vi "Teleop.vi"(10 "Match Info":T1={"Autonomous Elapsed Seconds"=0.0, "TeleOp Elapsed Seconds"=0.0, "Disabled Elapsed Seconds"=0.0, "Visited Autonomous"=FALSE, "Visited TeleOp"=FALSE, "Visited Disabled"=FALSE, "Autonomous Settings"={"Autonomous Style"=enum."Independent", "VI Refnum"=refnum}}, 11 "Call Context":T2) -> ()   [LabVIEW 2017]
doc: "This VI is called for each TeleOp packet received from the DS where the robot is not disabled. It is often used to read from the joysticks and update I/O or to update setpoints for timed control loops. It should complete and return within 20 milliseconds or it may miss DS packets."
uses:
  <vilib>/Rock Robotics/WPI/DriverStation/WPI_DriverStationDerivedRobotMode.ctl
  <vilib>/Rock Robotics/WPI/DriverStation/WPI_DriverStationMatch Info.ctl
  Public/Documents/Cross The Road Electronics/Phoenix-LabVIEW/Motor Controller/Controls/CTRE_Phoenix_MotorControl_ControlMode.ctl
  Public/Documents/Cross The Road Electronics/Phoenix-LabVIEW/Motor Controller/Controls/CTRE_Phoenix_MotorControl_FeedbackDevice.ctl
  <vilib>/Rock Robotics/Network Tables/NT Read Boolean.vi
  Public/Documents/Cross The Road Electronics/Phoenix-LabVIEW/Motor Controller/Get/CTRE_Phoenix_MotorController_GetSelectedSensorData.vi
  Public/Documents/Cross The Road Electronics/Phoenix-LabVIEW/Motor Controller/Get/CTRE_Phoenix_MotorController_GetPulseWidthAll.vi
  <vilib>/Utility/config.llb/Write Key (I32).vi
  <vilib>/Rock Robotics/Network Tables/NT Write Boolean.vi
  <vilib>/Utility/config.llb/Read Key (Double).vi
  <vilib>/Rock Robotics/Network Tables/NT Write Number.vi
  <vilib>/Rock Robotics/WPI/Utilities/WPI_GetSetVariantRefNum.vi
  Public/Documents/Cross The Road Electronics/Phoenix-LabVIEW/Motor Controller/Get/CTRE_Phoenix_MotorController_GetQuadratureData.vi
  <vilib>/Rock Robotics/WPI/Solenoid/Deprecated/WPI_SolenoidSetBool.vi
  Public/Documents/Cross The Road Electronics/Phoenix-LabVIEW/Motor Controller/Get/CTRE_Phoenix_MotorController_GetTemperature.vi
  Public/Documents/Cross The Road Electronics/Phoenix-LabVIEW/Motor Controller/Get/CTRE_Phoenix_MotorController_GetOutputCurrent_Enhanced.vi
  Robot Global Data.vi
  <vilib>/Utility/config.llb/NI_LVConfig.lvlib
  <vilib>/ptbypt/NI_PtbyPt.lvlib
panel:
  out "hasSet":bool
  out "ClimberDelay":dbl
  out "Holding Current":dbl=9001.0
  out "Old Direction":bool
  out "Stalled":bool
  out "OutHalf":bool
  out "EndGame":bool
  out "In":bool
  out "Hook":bool
  out "OutFULL":bool
  out "RobotOrientedPos":dbl
  out "RobotOriented":bool
  in  "Elevator Config":dbl(slide) scale=-1.0..1.0
  out "Rotate 3":dbl
  out "Rotate 2":dbl
  out "Rotate 1":dbl
  out "Rotate 0":dbl
  out "Turn3":dbl
  out "Turn2":dbl
  out "Turn1":dbl
  out "Turn0":dbl
  out "Speed0":dbl
  out "Speed1":dbl
  out "Speed2":dbl
  out "Speed3":dbl
  out "max":dbl
  out "angle":dbl
  out "temp":dbl
  out "Y":dbl
  out "X":dbl
  out "C":dbl
  out "D":dbl
  out "B":dbl
  out "A":dbl
  out "R":dbl
  out "W":dbl=22.75
  out "L":dbl=22.25
  out "RCW":dbl
  out "STR":dbl
  out "FWD":dbl
  out "Temp Speed0":dbl
  out "Temp Speed1":dbl
  out "Temp Speed2":dbl
  out "Temp Speed3":dbl
  out "Temp Turn3":dbl
  out "Temp Turn2":dbl
  out "Temp Turn1":dbl
  out "Temp Turn0":dbl
  out "Elevator Set":dbl=400.0
  out "Elevator Up":bool
  out "Elevator Pry":bool
  out "Elevator Middle":bool
  out "Elevator Down":bool
  out "Found 0? 2":bool
  out "Found 1? 2":bool
  out "Found 2? 2":bool
  out "Found 3? 2":bool
  out "Start Pos 7":i32
  out "Start Pos 6":i32
  out "Start Pos 5":i32
  out "Start Pos 4":i32
  in  "Read Button 2":bool
  out "Current Pos 7":i32
  out "Current Pos 6":i32
  out "Current Pos 5":i32
  out "Current Pos 4":i32
  out "Current Pos 3":i32
  out "Current Pos 1":i32
  out "Current Pos 2":i32
  out "Current Pos 0":i32
  out "Found 0?":bool
  out "Found 1?":bool
  out "Found 2?":bool
  out "Found 3?":bool
  in  "Write Button":bool
  out "Start Pos 3":i32
  out "Start Pos 2":i32
  out "Start Pos 1":i32
  out "Start Pos 0":i32
  in  "Read Button":bool
  out "0-4096 2":dbl
  out "Prev Knob Value":dbl
  out "Intake Motor":dbl
  in  "DriveMode":string(combo)="Mike1"
  out "0-4096":dbl
  out "+-180":dbl
  out "DegDir":dbl
  out "Elevator Change":bool
  out "Aquire":bool
  out "ArmLift":dbl
  out "Knob Value":dbl
  out "Arm Position":dbl
  out "Open/Close":bool
  out "Output Current":dbl
  out "Standby":bool
  out "StandbyWait":dbl
  out "Elevator Read":dbl
  out "Zero Gyro":bool
  out "TONY MODE":bool
  out "Direction":dbl
  out "DIAL":dbl
  out "Gyro":dbl
  out "Pos 3":i32
  out "Pos 2":i32
  out "Pos 1":i32
  out "Joystick":dbl
  out "Pos 0":i32
  out "Distance 2 Go":dbl
  out "Magnitude":dbl
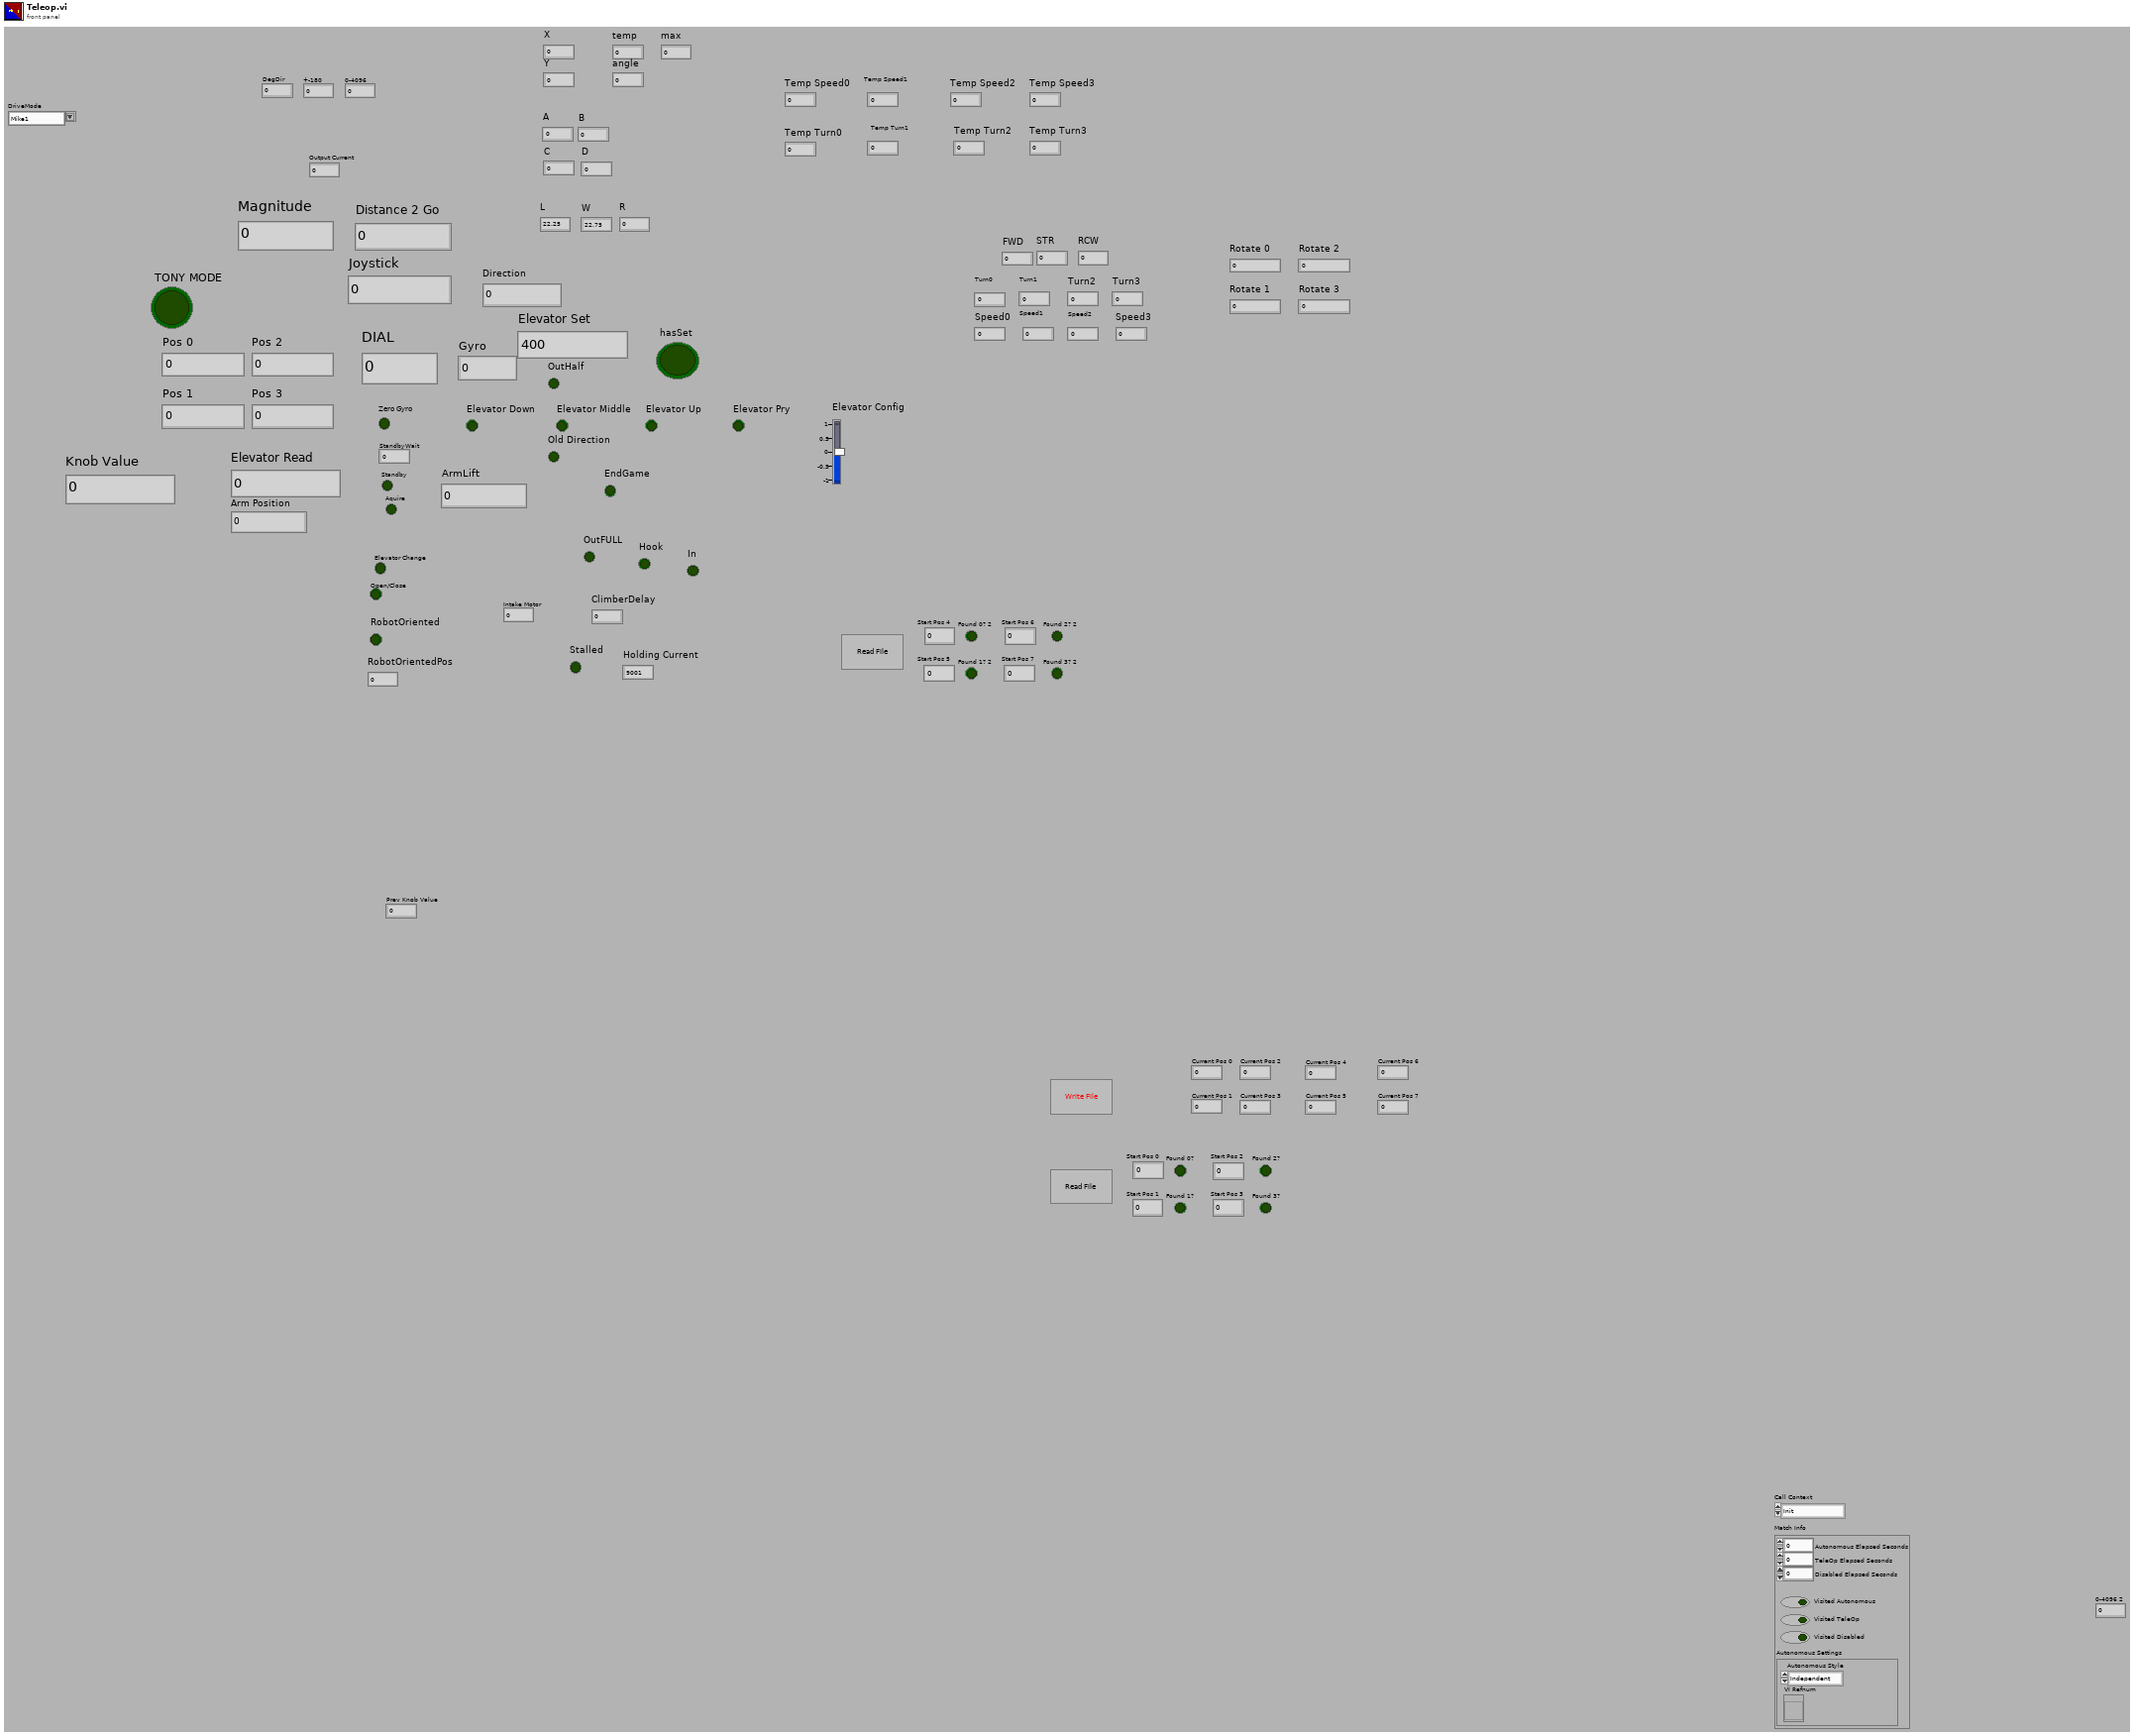
[diagram p1: front panel]
types:
  T1 = typedef "WPI_DriverStationMatch Info.ctl" = cluster{"Autonomous Elapsed Seconds":dbl, "TeleOp Elapsed Seconds":dbl, "Disabled Elapsed Seconds":dbl, "Visited Autonomous":bool, "Visited TeleOp":bool, "Visited Disabled":bool, "Autonomous Settings":cluster{"Autonomous Style":enum16{"Iterative", "Independent"}, "VI Refnum":refnum<vi>}}
  T2 = typedef "WPI_DriverStationDerivedRobotMode.ctl" = enum16{"Init", "Execute", "Stop"}
  T3 = typedef "CTRE_Phoenix_MotorControl_ControlMode.ctl" = u16
  T4 = typedef "WPI_MotorControlDeviceRef.ctl" = cluster{"DeviceStatus":errorcluster, "Type":T5, "PWM":cluster{"PWM Channel":T6, "DeadBand":T7}, "CAN":cluster{"Device Number":u8, "SetOutput VI Ref":variant, "GetOutput VI Ref":variant, "Enable VI Ref":variant, "Disable VI Ref":variant, "Data":variant}, "Invert":bool, "DIO PWM":cluster{"PWM \"Enable\" Channel":T6, "DIOChannel":T8, "PWM Rate":dbl}}
  T5 = typedef "WPI_MotorControlType.ctl" = enum16{"PWM", "CAN", "DIO PWM"}
  T6 = typedef "FPGA_DIOPWMChannel.ctl" = enum8{"PWM 0", "PWM 1", "PWM 2", "PWM 3", "PWM 4", "PWM 5", "PWM 6", "PWM 7", "PWM 8", "PWM 9", "PWM MXP 0", "PWM MXP 1", "PWM MXP 2", "PWM MXP 3", "PWM MXP 4", "PWM MXP 5", "PWM MXP 6", "PWM MXP 7", "PWM MXP 8", "PWM MXP 9", "Invalid"}
  T7 = typedef "WPI_PWMDeadband.ctl" = cluster{"Name":string, "maxPositivePwm":i32, "minPositivePwm":i32, "centerPwm":i32, "maxNegativePwm":i32, "minNegativePwm":i32, "angularRange":u16}
  T8 = typedef "FPGA_DIOChannel.ctl" = enum8{"DIO 0", "DIO 1", "DIO 2", "DIO 3", "DIO 4", "DIO 5", "DIO 6", "DIO 7", "DIO 8", "DIO 9", "DIO MXP 0", "DIO MXP 1", "DIO MXP 2", "DIO MXP 3", "DIO MXP 4", "DIO MXP 5", "DIO MXP 6", "DIO MXP 7", "DIO MXP 8", "DIO MXP 9", "DIO MXP 10", "DIO MXP 11", "DIO MXP 12", "DIO MXP 13", "DIO MXP 14", "DIO MXP 15", "SPI Port CS1", "SPI Port CS2", "SPI Port CS3", "SPI Port MISO", "SPI Port MOSI", "Invalid"}
  T9 = typedef "CTRE_Phoenix_MotorControl_FeedbackDevice.ctl" = i8
  T10 = typedef "NI_LVConfig.lvlib/Config Data RefNum.ctl" = refnum<k1>
  T11 = typedef "WPI_JoystickDevRef.ctl" = cluster{"Device":T12}
  T12 = typedef "WPI_JoystickDeviceEnum.ctl" = enum16{"USB 0", "USB 1", "USB 2", "USB 3", "USB 4", "USB 5"}
  T13 = typedef "WPI_CompressorDevRef.ctl" = cluster{"DevStatus":errorcluster, "Pneumatics Control Module":u8}
  T14 = typedef "WPI_SolenoidDevRef.ctl" = cluster{"DevStatus":errorcluster, "Pneumatics Control Module":u8, "Forward Solenoid Channel":T15, "Reverse Solenoid Channel":T15}
  T15 = typedef "WPI_SolenoidChannel.ctl" = enum8{"Solenoid 0", "Solenoid 1", "Solenoid 2", "Solenoid 3", "Solenoid 4", "Solenoid 5", "Solenoid 6", "Solenoid 7", "Invalid"}
  T16 = typedef "WPI_GyroDevRef.ctl" = cluster{"DevStatus":errorcluster, "Analog Channel":T17, "Gain (VoltsPerDegree/Second)":dbl, "Gyro Type":enum16{"Analog", "XRS450"}, "Handle":i32, "SPI Bus":T18, "Device Found":bool, "Sample Rate":dbl, "Calibrate On Open":bool, "Offset":dbl}
  T17 = typedef "FPGA_AIChannel.ctl" = enum8{"AI 0", "AI 1", "AI 2", "AI 3", "AI MXP 0", "AI MXP 1", "AI MXP 2", "AI MXP 3", "Invalid"}
  T18 = typedef "spi_bus.ctl" = enum16{"SPI On-Board, CS0", "SPI On-Board, CS1", "SPI On-Board, CS2", "SPI On-Board, CS3", "SPI MXP", "Invalid"}
  T19 = typedef "WPI_DigitalInputDevRef.ctl" = cluster{"DevStatus":errorcluster, "DIO Channel":T8}
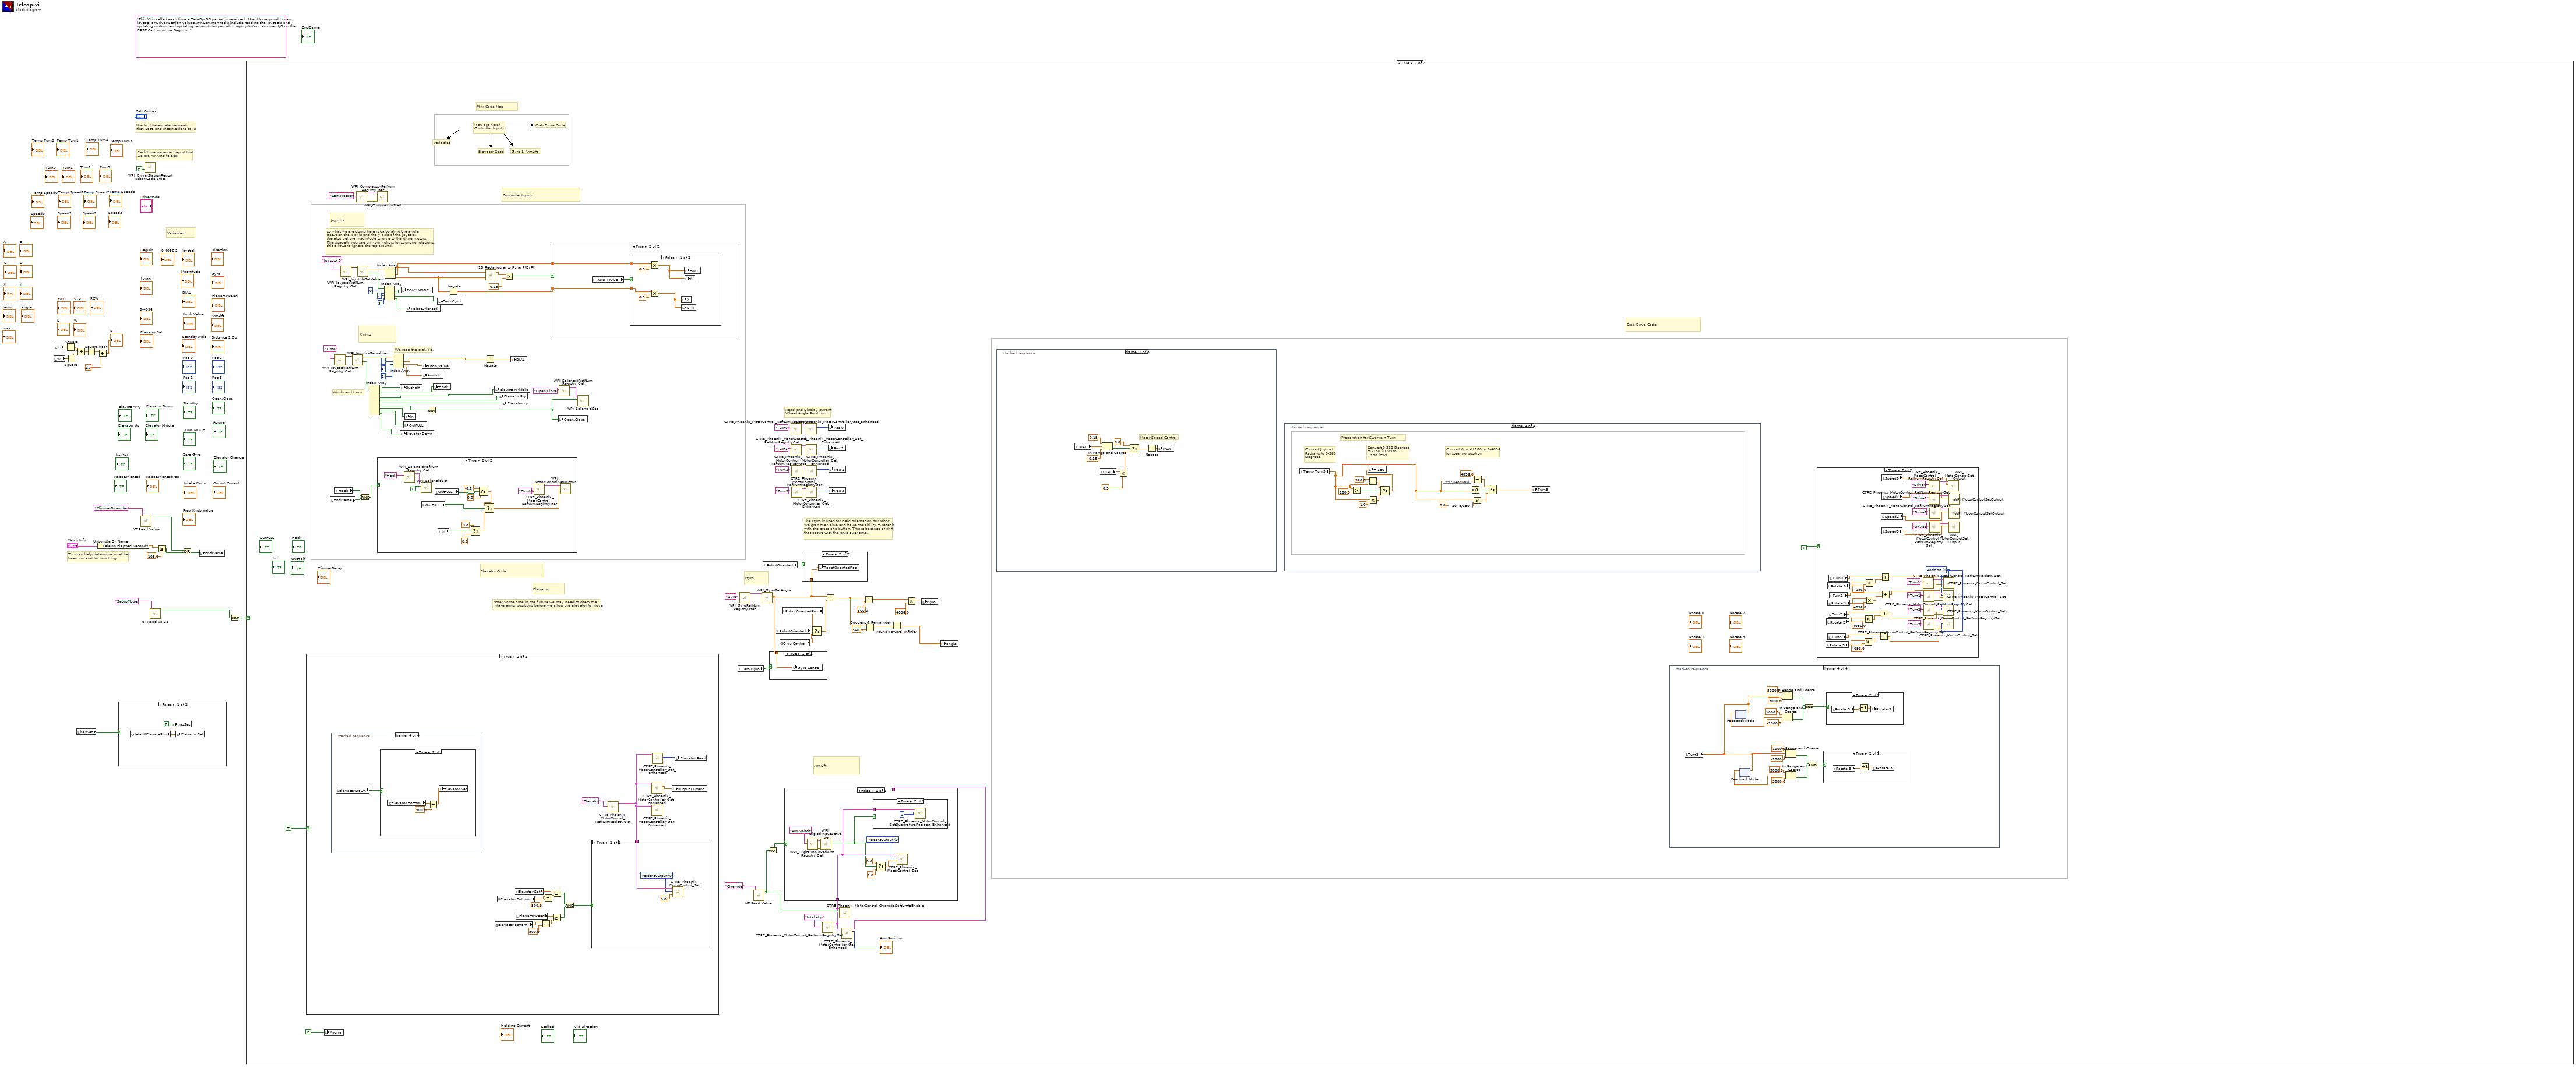
[diagram p0: block diagram]
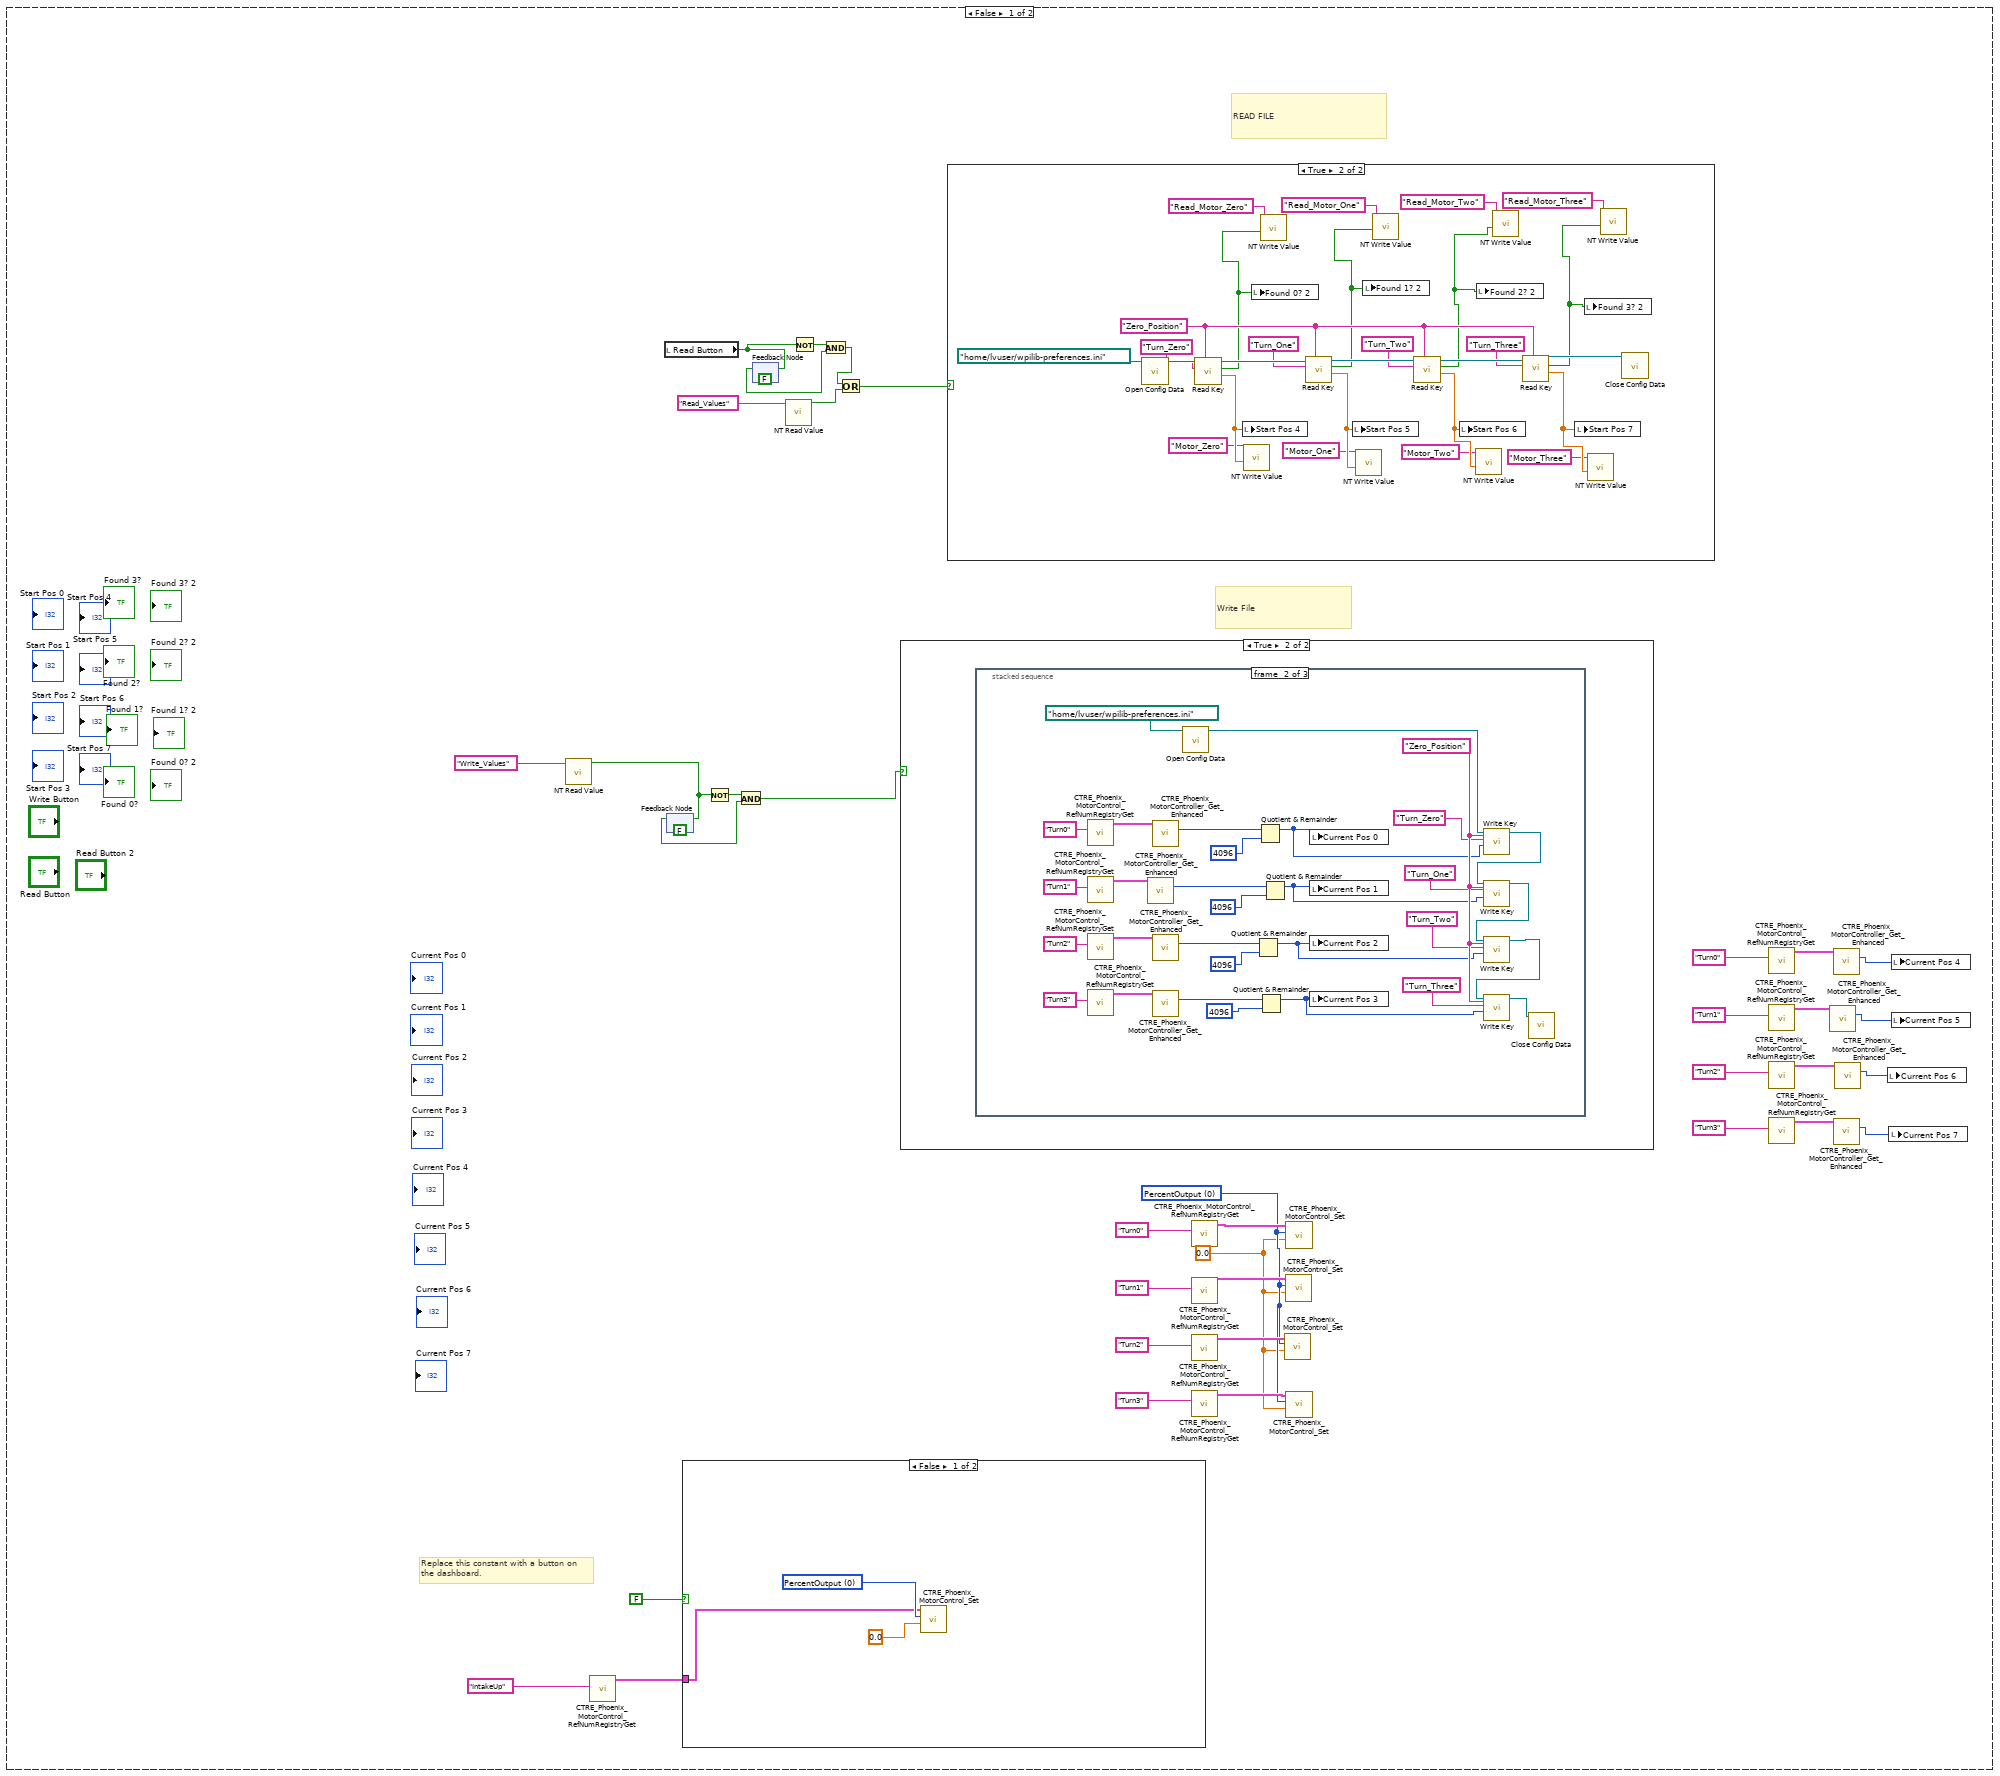
[diagram p3: hidden frame]
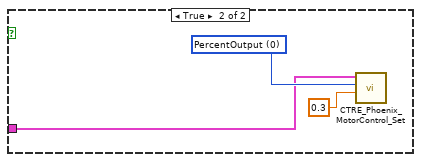
[diagram p4: hidden frame]
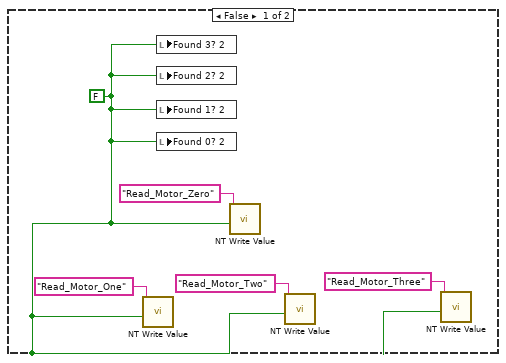
[diagram p5: hidden frame]
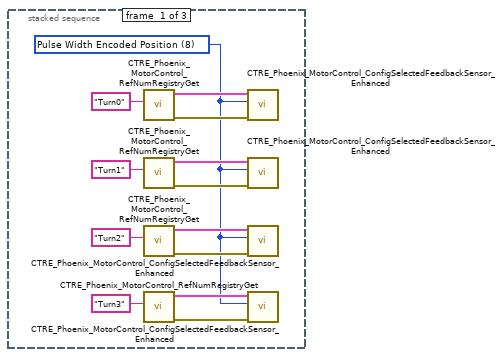
[diagram p7: hidden frame]
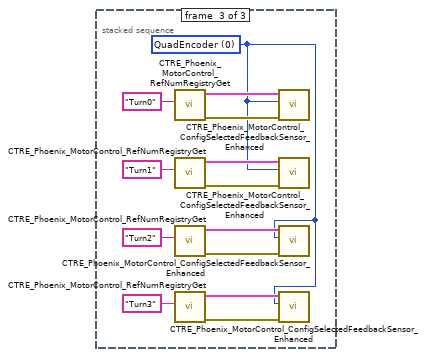
[diagram p8: hidden frame]
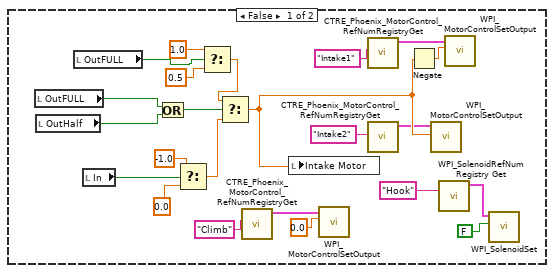
[diagram p9: hidden frame]
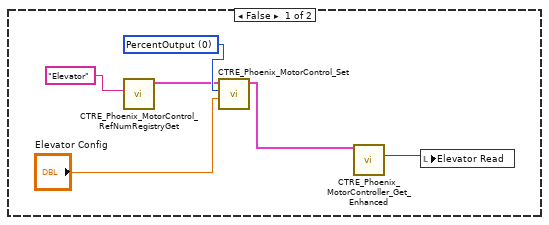
[diagram p11: hidden frame]
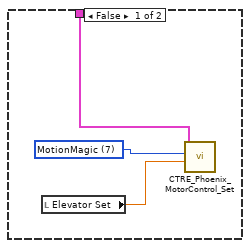
[diagram p12: hidden frame]
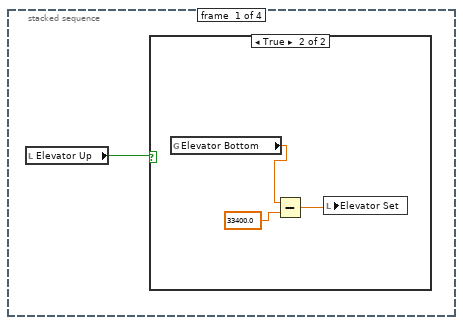
[diagram p13: hidden frame]
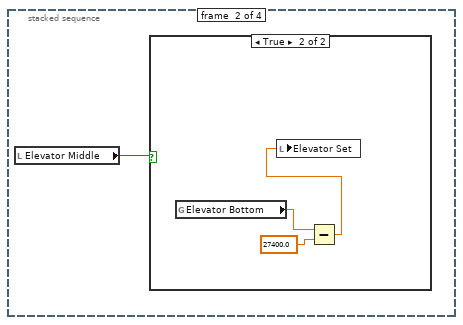
[diagram p15: hidden frame]
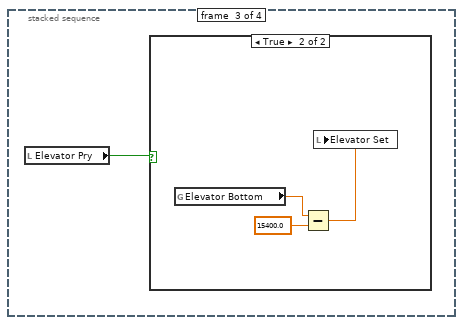
[diagram p17: hidden frame]
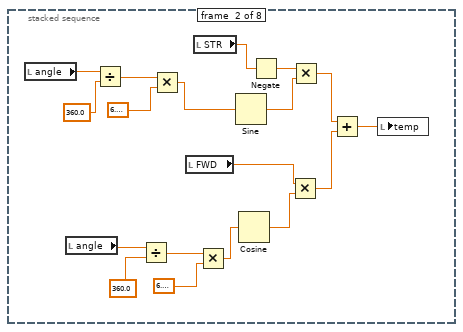
[diagram p20: hidden frame]
diagram:
  (unwired) "This VI is called each time a TeleOp DS packet is received.  Use it to respond to new joystick or Driver Station values.\n\nCommon tasks include reading the joysticks and updating motors, and updating setpoints for periodic loops.\n\nYou can open I/O on the FIRST Call, or in the Begin.vi."
  # "Each time we enter, report that\nwe are running teleop"
  # "Use to differentiate between\nFirst, Last, and Intermediate calls"
  # "This can help determine what has\nbeen run and for how long"
  # "Variables"
  n1 = local read "W"() -> (w14:dbl)
  n2 = local read "L"() -> (w15:dbl)
  n3 = Square(x=w15) -> (x^2=w13:dbl)
  n4 = Square(x=w14) -> (x^2=w11:dbl)
  n5 = Add(x=w13, y=w11) -> (x+y=w12:dbl)
  n6 = local read "hasSet"() -> (w1:bool)
  n7 = Square Root(x=w12) -> (sqrt(x)=w10:dbl)
  n8 = Divide(x=w10, y=2.0) -> (x/y=→"R":dbl)
  n9 = Unbundle By Name("Match Info") -> ("TeleOp Elapsed Seconds"=w7:dbl)
  n10 = case shown="False" w1 {
    frame False {
      n11 = global read "Robot Global Data.vi" "defaultElevatePos"() -> (w22:dbl)
      n12 = local write "hasSet"(TRUE ("hasSet")) -> ()
      n13 = local write "Elevator Set"(w22) -> ()
    }
    frame True {
    }
  }
  n14 = call-poly <vilib>:"NT Read Value.vi"("Name"="ClimberOverrider") -> ("Boolean"=w2:bool)  [unwired: 9 in, 1 out]
  n15 = call <vilib>:"WPI_DriverStationReport Robot Code State.vi"("TeleOp"=TRUE ("Autonomous")) -> ()  [unwired: 10 in, 1 out]
  n16 = call-poly <vilib>:"NT Read Value.vi"("Name"="SetupMode") -> ("Boolean"=w18:bool)  [unwired: 9 in, 1 out]
  n17 = Greater Or Equal?(x=w7, y=105.0) -> (x >= y?=w6:bool)
  n18 = Or(x=w2, y=w6) -> (x .or. y?=w3:bool)
  n19 = local write "EndGame"(w3) -> ()
  n20 = Not(x=w18) -> (.not. x?=w19:bool)
  n21 = case shown="True" w19 {
    frame False {
      w36 = 0.0 ("Output")
      w37 = T3 0 items=["PercentOutput"=0, "Position"=1, "Velocity"=2, "Current"=3, "Follower"=5, "MotionProfile"=6, "MotionMagic"=7, "MotionMagicArc"=8, "MotionProfileArc"=10, "Disabled"=15] ("Control Mode")
      # "Replace this constant with a button on\nthe dashboard."
      # "READ FILE"
      # "Write File"
      n22 = call-poly <vilib>:"NT Read Value.vi"("Name"="Write_Values") -> ("Boolean"=w34:bool)  [unwired: 9 in, 1 out]
      n23 = call "CTRE_Phoenix_MotorControl_RefNumRegistryGet.vi"("refnum name"="IntakeUp") -> ("PhoenixMotorControlDevRef"=w24:T4)  [unwired: 9 in, 1 out]
      n24 = local read "Read Button"() -> (w32:bool)
      n25 = feedback #1(FALSE ("Write Button")) -> (w59:bool)
      n26 = feedback-in #1(w34) -> ()
      n27 = case shown="False" FALSE {
        tunnel: w24 -> [w62 w66]
        frame False {
          w63 = T3 0 items=["PercentOutput"=0, "Position"=1, "Velocity"=2, "Current"=3, "Follower"=5, "MotionProfile"=6, "MotionMagic"=7, "MotionMagicArc"=8, "MotionProfileArc"=10, "Disabled"=15] ("Control Mode")
          n28 = call "CTRE_Phoenix_MotorControl_Set.vi"("Output"=0.0, "Control Mode"=w63, "PhoenixMotorControlDevRef"=w62) -> ()  [unwired: 7 in, 2 out]
        }
        frame True {
          w67 = T3 0 items=["PercentOutput"=0, "Position"=1, "Velocity"=2, "Current"=3, "Follower"=5, "MotionProfile"=6, "MotionMagic"=7, "MotionMagicArc"=8, "MotionProfileArc"=10, "Disabled"=15] ("Control Mode")
          n29 = call "CTRE_Phoenix_MotorControl_Set.vi"("Output"=0.3, "Control Mode"=w67, "PhoenixMotorControlDevRef"=w66) -> ()  [unwired: 7 in, 2 out]
        }
      }
      n30 = Not(x=w34) -> (.not. x?=w60:bool)
      n31 = And(x=w60, y=w59) -> (x .and. y?=w35:bool)
      n32 = feedback #2(FALSE ("Write Button")) -> (w31:bool)
      n33 = feedback-in #2(w32) -> ()
      n34 = call-poly <vilib>:"NT Read Value.vi"("Name"="Read_Values") -> ("Boolean"=w28:bool)  [unwired: 9 in, 1 out]
      n35 = Not(x=w32) -> (.not. x?=w30:bool)
      n36 = And(x=w30, y=w31) -> (x .and. y?=w33:bool)
      n37 = Or(x=w33, y=w28) -> (x .or. y?=w29:bool)
      n38 = case shown="True" w35 {
        frame False {
        }
        frame True {
          n39 = stacked-sequence {
            frame #0 {
              w100 = T9 8 items=["None"=-1, "QuadEncoder"=0, "Analog"=2, "Tachometer"=4, "Pulse Width Encoded Position"=8, "Sensor Sum (S0 + S1)"=9, "Sensor Difference (D0 - D1)"=10, "Remote Source 0"=11, "Remote Source 1"=12, "Software Emulated"=15] ("Feedback Device")
              n40 = call "CTRE_Phoenix_MotorControl_RefNumRegistryGet.vi"("refnum name"="Turn0") -> ("error out"=w108:errorcluster, "PhoenixMotorControlDevRef"=w107:T4)  [unwired: 9 in]
              n41 = call "CTRE_Phoenix_MotorControl_RefNumRegistryGet.vi"("refnum name"="Turn1") -> ("error out"=w106:errorcluster, "PhoenixMotorControlDevRef"=w105:T4)  [unwired: 9 in]
              n42 = call "CTRE_Phoenix_MotorControl_RefNumRegistryGet.vi"("refnum name"="Turn2") -> ("error out"=w104:errorcluster, "PhoenixMotorControlDevRef"=w103:T4)  [unwired: 9 in]
              n43 = call "CTRE_Phoenix_MotorControl_RefNumRegistryGet.vi"("refnum name"="Turn3") -> ("error out"=w102:errorcluster, "PhoenixMotorControlDevRef"=w101:T4)  [unwired: 9 in]
              n44 = call "CTRE_Phoenix_MotorControl_ConfigSelectedFeedbackSensor_Enhanced.vi"("error in (no error)"=w108, "Feedback Device"=w100, "PhoenixMotorControlDevRef"=w107) -> ()  [unwired: 7 in, 2 out]
              n45 = call "CTRE_Phoenix_MotorControl_ConfigSelectedFeedbackSensor_Enhanced.vi"("error in (no error)"=w106, "Feedback Device"=w100, "PhoenixMotorControlDevRef"=w105) -> ()  [unwired: 7 in, 2 out]
              n46 = call "CTRE_Phoenix_MotorControl_ConfigSelectedFeedbackSensor_Enhanced.vi"("error in (no error)"=w104, "Feedback Device"=w100, "PhoenixMotorControlDevRef"=w103) -> ()  [unwired: 7 in, 2 out]
              n47 = call "CTRE_Phoenix_MotorControl_ConfigSelectedFeedbackSensor_Enhanced.vi"("error in (no error)"=w102, "Feedback Device"=w100, "PhoenixMotorControlDevRef"=w101) -> ()  [unwired: 7 in, 2 out]
            }
            frame #1 {
              w138 = "Zero_Position" ("section")
              n48 = call "CTRE_Phoenix_MotorControl_RefNumRegistryGet.vi"("refnum name"="Turn0") -> ("PhoenixMotorControlDevRef"=w129:T4)  [unwired: 9 in, 1 out]
              n49 = call "CTRE_Phoenix_MotorControl_RefNumRegistryGet.vi"("refnum name"="Turn1") -> ("PhoenixMotorControlDevRef"=w130:T4)  [unwired: 9 in, 1 out]
              n50 = call "CTRE_Phoenix_MotorControl_RefNumRegistryGet.vi"("refnum name"="Turn2") -> ("PhoenixMotorControlDevRef"=w131:T4)  [unwired: 9 in, 1 out]
              n51 = call "CTRE_Phoenix_MotorControl_RefNumRegistryGet.vi"("refnum name"="Turn3") -> ("PhoenixMotorControlDevRef"=w132:T4)  [unwired: 9 in, 1 out]
              n52 = call-poly "CTRE_Phoenix_MotorController_Get_Enhanced.vi"("PhoenixMotorControlDevRef"=w130) -> ("Pulse Width Position"=w126:i32)  [unwired: 9 in, 5 out]
              n53 = call-poly "CTRE_Phoenix_MotorController_Get_Enhanced.vi"("PhoenixMotorControlDevRef"=w129) -> ("Pulse Width Position"=w125:i32)  [unwired: 9 in, 5 out]
              n54 = call-poly "CTRE_Phoenix_MotorController_Get_Enhanced.vi"("PhoenixMotorControlDevRef"=w132) -> ("Pulse Width Position"=w128:i32)  [unwired: 9 in, 5 out]
              n55 = call-poly "CTRE_Phoenix_MotorController_Get_Enhanced.vi"("PhoenixMotorControlDevRef"=w131) -> ("Pulse Width Position"=w127:i32)  [unwired: 9 in, 5 out]
              n56 = call <vilib>:"Open Config Data.vi"("configuration file path"=path "/home/lvuser/wpilib-preferences.ini") -> ("refnum"=w139:T10)  [unwired: 8 in, 2 out]
              n57 = Quotient & Remainder(x=w127, y=4096) -> (x-y*floor(x/y)=w114:i32)  [unwired: 1 out]
              n58 = Quotient & Remainder(x=w125, y=4096) -> (x-y*floor(x/y)=w116:i32)  [unwired: 1 out]
              n59 = Quotient & Remainder(x=w128, y=4096) -> (x-y*floor(x/y)=w113:i32)  [unwired: 1 out]
              n60 = Quotient & Remainder(x=w126, y=4096) -> (x-y*floor(x/y)=w115:i32)  [unwired: 1 out]
              n61 = local write "Current Pos 0"(w116) -> ()
              n62 = local write "Current Pos 1"(w115) -> ()
              n63 = local write "Current Pos 2"(w114) -> ()
              n64 = local write "Current Pos 3"(w113) -> ()
              n65 = call-poly <vilib>:"Write Key.vi"("section"=w138, "value"=w116, "key"="Turn_Zero", "refnum"=w139) -> ("refnum out"=w140:T10)  [unwired: 5 in, 2 out]
              n66 = call-poly <vilib>:"Write Key.vi"("section"=w138, "value"=w115, "key"="Turn_One", "refnum"=w140) -> ("refnum out"=w141:T10)  [unwired: 5 in, 2 out]
              n67 = call-poly <vilib>:"Write Key.vi"("section"=w138, "value"=w114, "key"="Turn_Two", "refnum"=w141) -> ("refnum out"=w142:T10)  [unwired: 5 in, 2 out]
              n68 = call-poly <vilib>:"Write Key.vi"("section"=w138, "value"=w113, "key"="Turn_Three", "refnum"=w142) -> ("refnum out"=w143:T10)  [unwired: 5 in, 2 out]
              n69 = call <vilib>:"Close Config Data.vi"("refnum"=w143) -> ()  [unwired: 9 in, 2 out]
            }
            frame #2 {
              w144 = T9 0 items=["None"=-1, "QuadEncoder"=0, "Analog"=2, "Tachometer"=4, "Pulse Width Encoded Position"=8, "Sensor Sum (S0 + S1)"=9, "Sensor Difference (D0 - D1)"=10, "Remote Source 0"=11, "Remote Source 1"=12, "Software Emulated"=15] ("Feedback Device")
              n70 = call "CTRE_Phoenix_MotorControl_RefNumRegistryGet.vi"("refnum name"="Turn0") -> ("error out"=w149:errorcluster, "PhoenixMotorControlDevRef"=w150:T4)  [unwired: 9 in]
              n71 = call "CTRE_Phoenix_MotorControl_RefNumRegistryGet.vi"("refnum name"="Turn1") -> ("error out"=w151:errorcluster, "PhoenixMotorControlDevRef"=w152:T4)  [unwired: 9 in]
              n72 = call "CTRE_Phoenix_MotorControl_RefNumRegistryGet.vi"("refnum name"="Turn2") -> ("error out"=w153:errorcluster, "PhoenixMotorControlDevRef"=w154:T4)  [unwired: 9 in]
              n73 = call "CTRE_Phoenix_MotorControl_RefNumRegistryGet.vi"("refnum name"="Turn3") -> ("error out"=w155:errorcluster, "PhoenixMotorControlDevRef"=w156:T4)  [unwired: 9 in]
              n74 = call "CTRE_Phoenix_MotorControl_ConfigSelectedFeedbackSensor_Enhanced.vi"("error in (no error)"=w149, "Feedback Device"=w144, "PhoenixMotorControlDevRef"=w150) -> ()  [unwired: 7 in, 2 out]
              n75 = call "CTRE_Phoenix_MotorControl_ConfigSelectedFeedbackSensor_Enhanced.vi"("error in (no error)"=w151, "Feedback Device"=w144, "PhoenixMotorControlDevRef"=w152) -> ()  [unwired: 7 in, 2 out]
              n76 = call "CTRE_Phoenix_MotorControl_ConfigSelectedFeedbackSensor_Enhanced.vi"("error in (no error)"=w153, "Feedback Device"=w144, "PhoenixMotorControlDevRef"=w154) -> ()  [unwired: 7 in, 2 out]
              n77 = call "CTRE_Phoenix_MotorControl_ConfigSelectedFeedbackSensor_Enhanced.vi"("error in (no error)"=w155, "Feedback Device"=w144, "PhoenixMotorControlDevRef"=w156) -> ()  [unwired: 7 in, 2 out]
            }
          }
        }
      }
      n78 = case shown="True" w29 {
        frame False {
          w68 = FALSE
          n79 = call-poly <vilib>:"NT Write Value.vi"("Boolean"=w68, "Name"="Read_Motor_One") -> ()  [unwired: 9 in, 1 out]
          n80 = local write "Found 3? 2"(w68) -> ()
          n81 = local write "Found 2? 2"(w68) -> ()
          n82 = local write "Found 1? 2"(w68) -> ()
          n83 = local write "Found 0? 2"(w68) -> ()
          n84 = call-poly <vilib>:"NT Write Value.vi"("Boolean"=w68, "Name"="Read_Motor_Zero") -> ()  [unwired: 9 in, 1 out]
          n85 = call-poly <vilib>:"NT Write Value.vi"("Boolean"=w68, "Name"="Read_Motor_Two") -> ()  [unwired: 9 in, 1 out]
          n86 = call-poly <vilib>:"NT Write Value.vi"("Boolean"=w68, "Name"="Read_Motor_Three") -> ()  [unwired: 9 in, 1 out]
        }
        frame True {
          w82 = "Zero_Position" ("section")
          n87 = call <vilib>:"Open Config Data.vi"("configuration file path"=path "/home/lvuser/wpilib-preferences.ini") -> ("refnum"=w99:T10)  [unwired: 8 in, 2 out]
          n88 = call-poly <vilib>:"Read Key.vi"("section"=w82, "key"="Turn_Zero", "refnum"=w99) -> ("value"=w94:dbl, "found?"=w73:bool, "refnum out"=w98:T10)  [unwired: 5 in, 1 out]
          n89 = local write "Start Pos 4"(w94) -> ()
          n90 = call-poly <vilib>:"NT Write Value.vi"("Numeric"=w94, "Name"="Motor_Zero") -> ()  [unwired: 9 in, 1 out]
          n91 = local write "Found 0? 2"(w73) -> ()
          n92 = call-poly <vilib>:"NT Write Value.vi"("Boolean"=w73, "Name"="Read_Motor_Zero") -> ()  [unwired: 9 in, 1 out]
          n93 = call-poly <vilib>:"Read Key.vi"("section"=w82, "key"="Turn_One", "refnum"=w98) -> ("value"=w93:dbl, "found?"=w74:bool, "refnum out"=w97:T10)  [unwired: 5 in, 1 out]
          n94 = local write "Start Pos 5"(w93) -> ()
          n95 = call-poly <vilib>:"NT Write Value.vi"("Numeric"=w93, "Name"="Motor_One") -> ()  [unwired: 9 in, 1 out]
          n96 = local write "Found 1? 2"(w74) -> ()
          n97 = call-poly <vilib>:"NT Write Value.vi"("Boolean"=w74, "Name"="Read_Motor_One") -> ()  [unwired: 9 in, 1 out]
          n98 = call-poly <vilib>:"Read Key.vi"("section"=w82, "key"="Turn_Two", "refnum"=w97) -> ("value"=w91:dbl, "found?"=w75:bool, "refnum out"=w96:T10)  [unwired: 5 in, 1 out]
          n99 = local write "Start Pos 6"(w91) -> ()
          n100 = call-poly <vilib>:"NT Write Value.vi"("Numeric"=w91, "Name"="Motor_Two") -> ()  [unwired: 9 in, 1 out]
          n101 = local write "Found 2? 2"(w75) -> ()
          n102 = call-poly <vilib>:"NT Write Value.vi"("Boolean"=w75, "Name"="Read_Motor_Two") -> ()  [unwired: 9 in, 1 out]
          n103 = call-poly <vilib>:"Read Key.vi"("section"=w82, "key"="Turn_Three", "refnum"=w96) -> ("value"=w92:dbl, "found?"=w76:bool, "refnum out"=w95:T10)  [unwired: 5 in, 1 out]
          n104 = local write "Start Pos 7"(w92) -> ()
          n105 = local write "Found 3? 2"(w76) -> ()
          n106 = call-poly <vilib>:"NT Write Value.vi"("Numeric"=w92, "Name"="Motor_Three") -> ()  [unwired: 9 in, 1 out]
          n107 = call-poly <vilib>:"NT Write Value.vi"("Boolean"=w76, "Name"="Read_Motor_Three") -> ()  [unwired: 9 in, 1 out]
          n108 = call <vilib>:"Close Config Data.vi"("refnum"=w95) -> ()  [unwired: 9 in, 2 out]
        }
      }
      n109 = call "CTRE_Phoenix_MotorControl_RefNumRegistryGet.vi"("refnum name"="Turn0") -> ("PhoenixMotorControlDevRef"=w41:T4)  [unwired: 9 in, 1 out]
      n110 = call "CTRE_Phoenix_MotorControl_RefNumRegistryGet.vi"("refnum name"="Turn1") -> ("PhoenixMotorControlDevRef"=w39:T4)  [unwired: 9 in, 1 out]
      n111 = call "CTRE_Phoenix_MotorControl_RefNumRegistryGet.vi"("refnum name"="Turn2") -> ("PhoenixMotorControlDevRef"=w40:T4)  [unwired: 9 in, 1 out]
      n112 = call "CTRE_Phoenix_MotorControl_RefNumRegistryGet.vi"("refnum name"="Turn3") -> ("PhoenixMotorControlDevRef"=w38:T4)  [unwired: 9 in, 1 out]
      n113 = call "CTRE_Phoenix_MotorControl_Set.vi"("Output"=w36, "Control Mode"=w37, "PhoenixMotorControlDevRef"=w40) -> ()  [unwired: 7 in, 2 out]
      n114 = call "CTRE_Phoenix_MotorControl_Set.vi"("Output"=w36, "Control Mode"=w37, "PhoenixMotorControlDevRef"=w39) -> ()  [unwired: 7 in, 2 out]
      n115 = call "CTRE_Phoenix_MotorControl_Set.vi"("Output"=w36, "Control Mode"=w37, "PhoenixMotorControlDevRef"=w41) -> ()  [unwired: 7 in, 2 out]
      n116 = call "CTRE_Phoenix_MotorControl_Set.vi"("Output"=w36, "Control Mode"=w37, "PhoenixMotorControlDevRef"=w38) -> ()  [unwired: 7 in, 2 out]
      n117 = call "CTRE_Phoenix_MotorControl_RefNumRegistryGet.vi"("refnum name"="Turn0") -> ("PhoenixMotorControlDevRef"=w46:T4)  [unwired: 9 in, 1 out]
      n118 = call "CTRE_Phoenix_MotorControl_RefNumRegistryGet.vi"("refnum name"="Turn1") -> ("PhoenixMotorControlDevRef"=w55:T4)  [unwired: 9 in, 1 out]
      n119 = call "CTRE_Phoenix_MotorControl_RefNumRegistryGet.vi"("refnum name"="Turn2") -> ("PhoenixMotorControlDevRef"=w56:T4)  [unwired: 9 in, 1 out]
      n120 = call "CTRE_Phoenix_MotorControl_RefNumRegistryGet.vi"("refnum name"="Turn3") -> ("PhoenixMotorControlDevRef"=w57:T4)  [unwired: 9 in, 1 out]
      n121 = call-poly "CTRE_Phoenix_MotorController_Get_Enhanced.vi"("PhoenixMotorControlDevRef"=w55) -> ("Position (Raw Sensor Units)"=w49:i32)  [unwired: 11 in, 3 out]
      n122 = call-poly "CTRE_Phoenix_MotorController_Get_Enhanced.vi"("PhoenixMotorControlDevRef"=w46) -> ("Position (Raw Sensor Units)"=w50:i32)  [unwired: 11 in, 3 out]
      n123 = call-poly "CTRE_Phoenix_MotorController_Get_Enhanced.vi"("PhoenixMotorControlDevRef"=w57) -> ("Position (Raw Sensor Units)"=w47:i32)  [unwired: 11 in, 3 out]
      n124 = call-poly "CTRE_Phoenix_MotorController_Get_Enhanced.vi"("PhoenixMotorControlDevRef"=w56) -> ("Position (Raw Sensor Units)"=w48:i32)  [unwired: 11 in, 3 out]
      n125 = local write "Current Pos 6"(w48) -> ()
      n126 = local write "Current Pos 7"(w47) -> ()
      n127 = local write "Current Pos 4"(w50) -> ()
      n128 = local write "Current Pos 5"(w49) -> ()
    }
    frame True {
      # "Crab Drive Code"
      # "Read and Display current\nWheel Angle Positions"
      # "ArmLift"
      # "Winch and Hook"
      # "Note: Some time in the furture we may need to check the \nintake arms' positions before we allow the elevator to move"
      # "Elevator"
      # "Gyro"
      # "Variables"
      # "Mini Code Map"
      # "Gyro & ArmLift"
      # "Elevator Code"
      # "Crab Drive Code"
      # "(You are here)\nController Inputs"
      # "Elevator Code"
      # "Controller Inputs"
      # "Xinmo"
      # "We read the dial. Ye."
      # "The Gyro is used for Field orientation our robot.\nWe grab the value and have the ability to reset it\nwith the press of a button. This is because of drift\nthat occurs with the gryo over time."
      # "so what we are doing here is calculating the angle\nbetween the x-axis and the y-axis of the joystick.\nWe also get the magnitude to give to the drive motors.\nThe spagetti you see on your right is for counting rotations,\nthis allows to ignore the rap-around."
      # "Joystick"
      n129 = case shown="True" TRUE {
        frame False {
          w285 = T3 0 items=["PercentOutput"=0, "Position"=1, "Velocity"=2, "Current"=3, "Follower"=5, "MotionProfile"=6, "MotionMagic"=7, "MotionMagicArc"=8, "MotionProfileArc"=10, "Disabled"=15] ("Control Mode")
          n130 = call "CTRE_Phoenix_MotorControl_RefNumRegistryGet.vi"("refnum name"="Elevator") -> ("PhoenixMotorControlDevRef"=w282:T4)  [unwired: 9 in, 1 out]
          n131 = call "CTRE_Phoenix_MotorControl_Set.vi"("Output"="Elevator Config", "Control Mode"=w285, "PhoenixMotorControlDevRef"=w282) -> ("PhoenixMotorControlDevRef"=w280:T4)  [unwired: 7 in, 1 out]
          n132 = call-poly "CTRE_Phoenix_MotorController_Get_Enhanced.vi"("PhoenixMotorControlDevRef"=w280) -> ("Pulse Width Position"=w281:i32)  [unwired: 9 in, 5 out]
          n133 = local write "Elevator Read"(w281) -> ()
        }
        frame True {
          n134 = stacked-sequence {
            frame #0 {
              n135 = local read "Elevator Up"() -> (w307:bool)
              n136 = case shown="True" w307 {
                frame False {
                }
                frame True {
                  n137 = global read "Robot Global Data.vi" "Elevator Bottom"() -> (w308:dbl)
                  n138 = Subtract(x=w308, y=33400.0 ("ElevatorScale")) -> (x-y=w309:dbl)
                  n139 = local write "Elevator Set"(w309) -> ()
                }
              }
            }
            frame #1 {
              n140 = local read "Elevator Middle"() -> (w311:bool)
              n141 = case shown="True" w311 {
                frame False {
                }
                frame True {
                  n142 = global read "Robot Global Data.vi" "Elevator Bottom"() -> (w313:dbl)
                  n143 = Subtract(x=w313, y=27400.0 ("ElevatorSwitch")) -> (x-y=w312:dbl)
                  n144 = local write "Elevator Set"(w312) -> ()
                }
              }
            }
            frame #2 {
              n145 = local read "Elevator Pry"() -> (w315:bool)
              n146 = case shown="True" w315 {
                frame False {
                }
                frame True {
                  n147 = global read "Robot Global Data.vi" "Elevator Bottom"() -> (w317:dbl)
                  n148 = Subtract(x=w317, y=15400.0) -> (x-y=w316:dbl)
                  n149 = local write "Elevator Set"(w316) -> ()
                }
              }
            }
            frame #3 {
              n150 = local read "Elevator Down"() -> (w319:bool)
              n151 = case shown="True" w319 {
                frame False {
                }
                frame True {
                  n152 = global read "Robot Global Data.vi" "Elevator Bottom"() -> (w322:dbl)
                  n153 = Subtract(x=w322, y=500.0) -> (x-y=w321:dbl)
                  n154 = local write "Elevator Set"(w321) -> ()
                }
              }
            }
          }
          n155 = global read "Robot Global Data.vi" "Elevator Bottom"() -> (w286:dbl)
          n156 = global read "Robot Global Data.vi" "Elevator Bottom"() -> (w290:dbl)
          n157 = local read "Elevator Set"() -> (w297:dbl)
          n158 = local read "Elevator Read"() -> (w296:dbl)
          n159 = Subtract(x=w286, y=500.0) -> (x-y=w287:dbl)
          n160 = Subtract(x=w290, y=500.0) -> (x-y=w291:dbl)
          n161 = Greater Or Equal?(x=w296, y=w287) -> (x >= y?=w293:bool)
          n162 = Equal?(x=w297, y=w291) -> (x = y?=w294:bool)
          n163 = And(x=w294, y=w293) -> (x .and. y?=w292:bool)
          n164 = call "CTRE_Phoenix_MotorControl_RefNumRegistryGet.vi"("refnum name"="Elevator") -> ("PhoenixMotorControlDevRef"=w295:T4)  [unwired: 9 in, 1 out]
          n165 = case shown="True" w292 {
            tunnel: w295 -> [w301 w306]
            frame False {
              w302 = T3 7 items=["PercentOutput"=0, "Position"=1, "Velocity"=2, "Current"=3, "Follower"=5, "MotionProfile"=6, "MotionMagic"=7, "MotionMagicArc"=8, "MotionProfileArc"=10, "Disabled"=15] ("Control Mode")
              n166 = local read "Elevator Set"() -> (w303:dbl)
              n167 = call "CTRE_Phoenix_MotorControl_Set.vi"("Output"=w303, "Control Mode"=w302, "PhoenixMotorControlDevRef"=w301) -> ()  [unwired: 7 in, 2 out]
            }
            frame True {
              w305 = T3 0 items=["PercentOutput"=0, "Position"=1, "Velocity"=2, "Current"=3, "Follower"=5, "MotionProfile"=6, "MotionMagic"=7, "MotionMagicArc"=8, "MotionProfileArc"=10, "Disabled"=15] ("Control Mode")
              n168 = call "CTRE_Phoenix_MotorControl_Set.vi"("Output"=0.0, "Control Mode"=w305, "PhoenixMotorControlDevRef"=w306) -> ()  [unwired: 7 in, 2 out]
            }
          }
          n169 = call-poly "CTRE_Phoenix_MotorController_Get_Enhanced.vi"("PhoenixMotorControlDevRef"=w295) -> ("Output Current"=w298:dbl)  [unwired: 12 in, 2 out]
          n170 = call-poly "CTRE_Phoenix_MotorController_Get_Enhanced.vi"("PhoenixMotorControlDevRef"=w295) -> ()  [unwired: 12 in, 3 out]
          n171 = call-poly "CTRE_Phoenix_MotorController_Get_Enhanced.vi"("PhoenixMotorControlDevRef"=w295) -> ("Pulse Width Position"=w299:i32)  [unwired: 9 in, 5 out]
          n172 = local write "Output Current"(w298) -> ()
          n173 = local write "Elevator Read"(w299) -> ()
        }
      }
      n174 = local write "Aquire"(FALSE) -> ()
      n175 = local read "EndGame"() -> (w159:bool)
      n176 = call <vilib>:"WPI_JoystickRefNum Registry Get.vi"("refnum name"="Ximo") -> ("JoystickDevRef"=w232:T11)  [unwired: 1 in, 9 out]
      n177 = local read "Hook"() -> (w160:bool)
      n178 = call <vilib>:"WPI_JoystickRefNum Registry Get.vi"("refnum name"="Joystick 0") -> ("JoystickDevRef"=w239:T11)  [unwired: 1 in, 9 out]
      n179 = call <vilib>:"WPI_JoystickGetValues.vi"("JoystickDevRef"=w232) -> ("Buttons"=w216:bool[], "Axes"=w233:dbl[])  [unwired: 6 in, 3 out]
      n180 = call <vilib>:"WPI_CompressorRefNum Registry Get.vi"("refnum name"="Compressor") -> ("error out"=w218:errorcluster, "CompressorDevRef"=w217:T13)  [unwired: 9 in]
      n181 = call <vilib>:"WPI_JoystickGetValues.vi"("JoystickDevRef"=w239) -> ("Buttons"=w229:bool[], "Axes"=w238:dbl[])  [unwired: 6 in, 3 out]
      n182 = And(x=w160, y=w159) -> (x .and. y?=w158:bool)
      n183 = Index Array(array=w216) -> (element #1=w162:bool, element #2=w161:bool, element #3=w175:bool, element #4=w174:bool, element #5=w192:bool, element #6=w215:bool, element #7=w164:bool, element #8=w163:bool, element #9=w191:bool)  [unwired: 9 in]
      n184 = call <vilib>:"WPI_CompressorStart.vi"("error in (no error)"=w218, "CompressorDevRef"=w217) -> ()  [unwired: 8 in, 2 out]
      n185 = case shown="True" w158 {
        frame False {
          n186 = local read "OutFULL"() -> (w260:bool)
          n187 = local read "OutHalf"() -> (w261:bool)
          n188 = local read "OutFULL"() -> (w263:bool)
          n189 = local read "In"() -> (w258:bool)
          n190 = Or(x=w260, y=w261) -> (x .or. y?=w262:bool)
          n191 = Select(t=-1.0, s=w258, f=0.0) -> (s? t:f=w255:dbl)
          n192 = Select(t=1.0, s=w263, f=0.5) -> (s? t:f=w259:dbl)
          n193 = Select(t=w259, s=w262, f=w255) -> (s? t:f=w257:dbl)
          n194 = call "CTRE_Phoenix_MotorControl_RefNumRegistryGet.vi"("refnum name"="Climb") -> ("PhoenixMotorControlDevRef"=w243:T4)  [unwired: 9 in, 1 out]
          n195 = local write "Intake Motor"(w257) -> ()
          n196 = call <vilib>:"WPI_MotorControlSetOutput.vi"("Output"=0.0, "MotorControlDevRef"=w243) -> ()  [unwired: 7 in, 3 out]
          n197 = call "CTRE_Phoenix_MotorControl_RefNumRegistryGet.vi"("refnum name"="Intake1") -> ("PhoenixMotorControlDevRef"=w253:T4)  [unwired: 9 in, 1 out]
          n198 = call "CTRE_Phoenix_MotorControl_RefNumRegistryGet.vi"("refnum name"="Intake2") -> ("PhoenixMotorControlDevRef"=w254:T4)  [unwired: 9 in, 1 out]
          n199 = Negate(x=w257) -> (-x=w256:dbl)
          n200 = call <vilib>:"WPI_MotorControlSetOutput.vi"("Output"=w257, "MotorControlDevRef"=w254) -> ()  [unwired: 7 in, 3 out]
          n201 = call <vilib>:"WPI_SolenoidRefNum Registry Get.vi"("refnum name"="Hook") -> ("SolenoidDevRef"=w246:T14)  [unwired: 9 in, 1 out]
          n202 = call <vilib>:"WPI_MotorControlSetOutput.vi"("Output"=w256, "MotorControlDevRef"=w253) -> ()  [unwired: 7 in, 3 out]
          n203 = call-poly <vilib>:"WPI_SolenoidSet.vi"("Value"=FALSE, "SolenoidDevRef"=w246) -> ()  [unwired: 8 in, 2 out]
        }
        frame True {
          n204 = call <vilib>:"WPI_SolenoidRefNum Registry Get.vi"("refnum name"="Hook") -> ("SolenoidDevRef"=w278:T14)  [unwired: 9 in, 1 out]
          n205 = call-poly <vilib>:"WPI_SolenoidSet.vi"("Value"=TRUE, "SolenoidDevRef"=w278) -> ()  [unwired: 8 in, 2 out]
          n206 = local read "OutFULL"() -> (w264:bool)
          n207 = local read "OutFULL"() -> (w275:bool)
          n208 = local read "In"() -> (w273:bool)
          n209 = Select(t=0.8, s=w273, f=0.0) -> (s? t:f=w271:dbl)
          n210 = Select(t=-0.2, s=w275, f=0.0) -> (s? t:f=w274:dbl)
          n211 = Select(t=w274, s=w264, f=w271) -> (s? t:f=w272:dbl)
          n212 = call "CTRE_Phoenix_MotorControl_RefNumRegistryGet.vi"("refnum name"="Climb") -> ("PhoenixMotorControlDevRef"=w270:T4)  [unwired: 9 in, 1 out]
          n213 = call <vilib>:"WPI_MotorControlSetOutput.vi"("Output"=w272, "MotorControlDevRef"=w270) -> ()  [unwired: 7 in, 3 out]
        }
      }
      n214 = Index Array(array=w229, index #1=0 ("index"), index #2=2 ("index"), index #3=3 ("index")) -> (element #1=w228:bool, element #2=w225:bool, element #3=w172:bool)
      n215 = Index Array(array=w238) -> (element #1=w179:dbl, element #2=w181:dbl)  [unwired: 2 in]
      n216 = Index Array(array=w233, index #1=4 ("index"), index #2=3 ("index"), index #3=1 ("index")) -> (element #1=w177:dbl, element #2=w211:dbl, element #3=w209:dbl)
      n217 = local write "OutHalf"(w161) -> ()
      n218 = local write "Elevator Down"(w191) -> ()
      n219 = local write "TONY MODE"(w228) -> ()
      n220 = local write "OutFULL"(w163) -> ()
      n221 = local write "In"(w164) -> ()
      n222 = local write "RobotOriented"(w172) -> ()
      n223 = local write "Knob Value"(w211) -> ()
      n224 = local write "ArmLift"(w209) -> ()
      n225 = Not(x=w215) -> (.not. x?=w198:bool)
      n226 = local write "Hook"(w162) -> ()
      n227 = local write "Zero Gyro"(w225) -> ()
      n228 = Negate(x=w181) -> (-x=w178:dbl)
      n229 = Negate(x=w177) -> (-x=w157:dbl)
      n230 = call <vilib>:"1D Rectangular to Polar PtByPt.vi"("y"=w181, "x"=w179) -> ("magnitude"=w196:dbl)  [unwired: 1 out]
      n231 = local write "Elevator Middle"(w175) -> ()
      n232 = local write "Elevator Pry"(w174) -> ()
      n233 = local write "Elevator Up"(w192) -> ()
      n234 = Greater?(x=w196, y=0.15) -> (0:w194:bool)
      n235 = local write "DIAL"(w157) -> ()
      n236 = case shown="True" w194 {
        tunnel: w179 -> [_ w602]
        tunnel: w178 -> [_ w601]
        frame False {
          w600 = 0.0 ("Y")
          n237 = local write "RCW"(w600) -> ()
          n238 = local write "X"(w600) -> ()
          n239 = local write "Y"(w600) -> ()
          n240 = local write "FWD"(w600) -> ()
          n241 = local write "STR"(w600) -> ()
        }
        frame True {
          n242 = local read "TONY MODE"() -> (w603:bool)
          n243 = case shown="False" w603 {
            tunnel: w602 -> [w609 w611]
            tunnel: w601 -> [w606 w610]
            frame False {
              n244 = Multiply(x=w609, y=0.5) -> (x*y=w604:dbl)
              n245 = Multiply(x=w606, y=0.5) -> (x*y=w605:dbl)
              n246 = local write "X"(w605) -> ()
              n247 = local write "STR"(w605) -> ()
              n248 = local write "FWD"(w604) -> ()
              n249 = local write "Y"(w604) -> ()
            }
            frame True {
              n250 = local write "Y"(w611) -> ()
              n251 = local write "X"(w610) -> ()
              n252 = local write "STR"(w610) -> ()
              n253 = local write "FWD"(w611) -> ()
            }
          }
        }
      }
      n254 = local write "Open/Close"(w198) -> ()
      n255 = call <vilib>:"WPI_SolenoidRefNum Registry Get.vi"("refnum name"="Open/Close") -> ("SolenoidDevRef"=w220:T14)  [unwired: 9 in, 1 out]
      n256 = call-poly <vilib>:"WPI_SolenoidSet.vi"("Value"=w198, "SolenoidDevRef"=w220) -> ()  [unwired: 8 in, 2 out]
      n257 = local read "Zero Gyro"() -> (w223:bool)
      n258 = call <vilib>:"WPI_GyroRefNum Registry Get.vi"("refnum name"="Gyro") -> ("GyroDevRef"=w234:T16)  [unwired: 9 in, 1 out]
      n259 = call-poly <vilib>:"NT Read Value.vi"("Name"="Override") -> ("Boolean"=w205:bool)  [unwired: 9 in, 1 out]
      n260 = call <vilib>:"WPI_GyroGetAngle.vi"("GyroDevRef"=w234) -> ("Angle"=w170:dbl)  [unwired: 6 in, 4 out]
      n261 = local read "RobotOriented"() -> (w171:bool)
      n262 = Not(x=w205) -> (.not. x?=w207:bool)
      n263 = case shown="True" w223 {
        tunnel: w170 -> [_ w707]
        frame False {
        }
        frame True {
          n264 = global write "Robot Global Data.vi" "Gyro Centre"(w707) -> ()
        }
      }
      n265 = local read "RobotOriented"() -> (w166:bool)
      n266 = global read "Robot Global Data.vi" "Gyro Centre"() -> (w169:dbl)
      n267 = local read "RobotOrientedPos"() -> (w168:dbl)
      n268 = call "CTRE_Phoenix_MotorControl_RefNumRegistryGet.vi"("refnum name"="Turn0") -> ("PhoenixMotorControlDevRef"=w236:T4)  [unwired: 9 in, 1 out]
      n269 = call "CTRE_Phoenix_MotorControl_RefNumRegistryGet.vi"("refnum name"="Turn1") -> ("PhoenixMotorControlDevRef"=w204:T4)  [unwired: 9 in, 1 out]
      n270 = call "CTRE_Phoenix_MotorControl_RefNumRegistryGet.vi"("refnum name"="Turn2") -> ("PhoenixMotorControlDevRef"=w201:T4)  [unwired: 9 in, 1 out]
      n271 = call "CTRE_Phoenix_MotorControl_RefNumRegistryGet.vi"("refnum name"="Turn3") -> ("PhoenixMotorControlDevRef"=w200:T4)  [unwired: 9 in, 1 out]
      n272 = case shown="True" w171 {
        tunnel: w170 -> [_ w279]
        frame False {
        }
        frame True {
          n273 = local write "RobotOrientedPos"(w279) -> ()
        }
      }
      n274 = call-poly "CTRE_Phoenix_MotorController_Get_Enhanced.vi"("PhoenixMotorControlDevRef"=w236) -> ("Quadrature Position"=w190:i32)  [unwired: 11 in, 3 out]
      n275 = call-poly "CTRE_Phoenix_MotorController_Get_Enhanced.vi"("PhoenixMotorControlDevRef"=w204) -> ("Quadrature Position"=w189:i32)  [unwired: 11 in, 3 out]
      n276 = call-poly "CTRE_Phoenix_MotorController_Get_Enhanced.vi"("PhoenixMotorControlDevRef"=w201) -> ("Quadrature Position"=w188:i32)  [unwired: 11 in, 3 out]
      n277 = call-poly "CTRE_Phoenix_MotorController_Get_Enhanced.vi"("PhoenixMotorControlDevRef"=w200) -> ("Quadrature Position"=w187:i32)  [unwired: 11 in, 3 out]
      n278 = Select(t=w168, s=w166, f=w169) -> (s? t:f=w167:dbl)
      n279 = call "CTRE_Phoenix_MotorControl_RefNumRegistryGet.vi"("refnum name"="IntakeUp") -> ("PhoenixMotorControlDevRef"=w176:T4)  [unwired: 9 in, 1 out]
      n280 = Subtract(x=w170, y=w167) -> (x-y=w184:dbl)
      n281 = local write "Pos 0"(w190) -> ()
      n282 = local write "Pos 1"(w189) -> ()
      n283 = local write "Pos 2"(w188) -> ()
      n284 = local write "Pos 3"(w187) -> ()
      n285 = call "CTRE_Phoenix_MotorControl_OverrideSoftLimtsEnable.vi"("PhoenixMotorControlDevRef"=w176, "Override Soft Limit Enable?"=w205) -> ()  [unwired: 12 in, 2 out]
      n286 = call-poly "CTRE_Phoenix_MotorController_Get_Enhanced.vi"("PhoenixMotorControlDevRef"=w176) -> ("PhoenixMotorControlDevRef"=w208:T4, "Quadrature Position"=→"Arm Position":i32)  [unwired: 11 in, 2 out]
      n287 = case shown="False" w207 {
        tunnel: w208 -> [_ w687]
        tunnel: w176 -> [w677 _]
        frame False {
          w684 = T3 0 items=["PercentOutput"=0, "Position"=1, "Velocity"=2, "Current"=3, "Follower"=5, "MotionProfile"=6, "MotionMagic"=7, "MotionMagicArc"=8, "MotionProfileArc"=10, "Disabled"=15] ("Control Mode")
          n288 = call <vilib>:"WPI_DigitalInputRefNum Registry Get.vi"("refnum name"="ArmSwitch") -> ("error out"=w682:errorcluster, "DigitalInputDevRef"=w681:T19)  [unwired: 9 in]
          n289 = call <vilib>:"WPI_DigitalInputGetValue.vi"("error in (no error)"=w682, "DigitalInputDevRef"=w681) -> ("Value"=w676:bool)  [unwired: 7 in, 2 out]
          n290 = case shown="True" w676 {
            tunnel: w677 -> [_ w686]
            frame False {
            }
            frame True {
              n291 = call <vilib>:"CTRE_Phoenix_MotorControl_SetQuadraturePosition_Enhanced.vi"("New Position"=0 ("New Sensor Position"), "PhoenixMotorControlDevRef"=w686) -> ()  [unwired: 8 in, 2 out]
            }
          }
          n292 = Select(t=0.0, s=w676, f=1.0) -> (s? t:f=w678:dbl)
          n293 = call "CTRE_Phoenix_MotorControl_Set.vi"("Output"=w678, "Control Mode"=w684, "PhoenixMotorControlDevRef"=w677) -> ()  [unwired: 7 in, 2 out]
        }
        frame True {
          n294 = local read "ArmLift"() -> (w691:dbl)
          n295 = In Range and Coerce(upper limit=1.1, x=w691, lower limit=0.75) -> (In Range?=w689:bool)  [unwired: 1 out]
          n296 = In Range and Coerce(upper limit=0.75, x=w691, lower limit=-0.75) -> (In Range?=w690:bool)  [unwired: 1 out]
          n297 = In Range and Coerce(upper limit=-0.75, x=w691, lower limit=-1.1) -> (In Range?=w688:bool)  [unwired: 1 out]
          n298 = case shown="True" w690 {
            tunnel: w687 -> [_ w702]
            frame False {
            }
            frame True {
              w701 = T3 1 items=["PercentOutput"=0, "Position"=1, "Velocity"=2, "Current"=3, "Follower"=5, "MotionProfile"=6, "MotionMagic"=7, "MotionMagicArc"=8, "MotionProfileArc"=10, "Disabled"=15] ("Control Mode")
              n299 = call "CTRE_Phoenix_MotorControl_Set.vi"("Output"=-2000.0, "Control Mode"=w701, "PhoenixMotorControlDevRef"=w702) -> ()  [unwired: 7 in, 2 out]
            }
          }
          n300 = case shown="True" w688 {
            tunnel: w687 -> [_ w699]
            frame False {
            }
            frame True {
              w698 = T3 1 items=["PercentOutput"=0, "Position"=1, "Velocity"=2, "Current"=3, "Follower"=5, "MotionProfile"=6, "MotionMagic"=7, "MotionMagicArc"=8, "MotionProfileArc"=10, "Disabled"=15] ("Control Mode")
              n301 = call "CTRE_Phoenix_MotorControl_Set.vi"("Output"=-4500.0, "Control Mode"=w698, "PhoenixMotorControlDevRef"=w699) -> ()  [unwired: 7 in, 2 out]
            }
          }
          n302 = case shown="True" w689 {
            tunnel: w687 -> [_ w706]
            frame False {
            }
            frame True {
              w705 = T3 1 items=["PercentOutput"=0, "Position"=1, "Velocity"=2, "Current"=3, "Follower"=5, "MotionProfile"=6, "MotionMagic"=7, "MotionMagicArc"=8, "MotionProfileArc"=10, "Disabled"=15] ("Control Mode")
              n303 = call "CTRE_Phoenix_MotorControl_Set.vi"("Output"=0.0, "Control Mode"=w705, "PhoenixMotorControlDevRef"=w706) -> ()  [unwired: 7 in, 2 out]
            }
          }
        }
      }
      n304 = Divide(x=w184, y=360.0) -> (x/y=w186:dbl)
      n305 = Quotient & Remainder(x=w184, y=360.0) -> (x-y*floor(x/y)=w183:dbl)  [unwired: 1 out]
      n306 = Round Toward -Infinity(1:w183) -> (0:w182:dbl)
      n307 = Multiply(x=w186, y=4096.0) -> (x*y=w222:dbl)
      n308 = local write "Gyro"(w222) -> ()
      n309 = local write "angle"(w182) -> ()
      n310 = stacked-sequence {
        frame #0 {
          # "Motor Speed Control"
          n311 = local read "DIAL"() -> (w331:dbl)
          n312 = local read "DIAL"() -> (w329:dbl)
          n313 = In Range and Coerce(upper limit=0.15, x=w331, lower limit=-0.15) -> (In Range?=w330:bool)  [unwired: 1 out]
          n314 = Multiply(x=w329, y=0.5) -> (x*y=w324:dbl)
          n315 = Select(t=0.0, s=w330, f=w324) -> (s? t:f=w332:dbl)
          n316 = Negate(x=w332) -> (-x=w325:dbl)
          n317 = local write "RCW"(w325) -> ()
        }
        frame #1 {
          n318 = local read "angle"() -> (w337:dbl)
          n319 = local read "angle"() -> (w344:dbl)
          n320 = Divide(x=w337, y=360.0) -> (x/y=w339:dbl)
          n321 = Divide(x=w344, y=360.0) -> (x/y=w341:dbl)
          n322 = Multiply(x=w339, y=6.283185307179586) -> (x*y=w335:dbl)
          n323 = local read "FWD"() -> (w334:dbl)
          n324 = local read "STR"() -> (w345:dbl)
          n325 = Multiply(x=w341, y=6.283185307179586) -> (x*y=w340:dbl)
          n326 = Sine(x=w335) -> (sin(x)=w350:dbl)
          n327 = Cosine(x=w340) -> (cos(x)=w349:dbl)
          n328 = Negate(x=w345) -> (-x=w333:dbl)
          n329 = Multiply(x=w334, y=w349) -> (x*y=w347:dbl)
          n330 = Multiply(x=w333, y=w350) -> (x*y=w346:dbl)
          n331 = Add(x=w346, y=w347) -> (x+y=w348:dbl)
          n332 = local write "temp"(w348) -> ()
        }
        frame #2 {
          n333 = local read "angle"() -> (w362:dbl)
          n334 = local read "angle"() -> (w356:dbl)
          n335 = Divide(x=w362, y=360.0) -> (x/y=w363:dbl)
          n336 = Divide(x=w356, y=360.0) -> (x/y=w355:dbl)
          n337 = Multiply(x=w363, y=6.283185307179586) -> (x*y=w359:dbl)
          n338 = Multiply(x=w355, y=6.283185307179586) -> (x*y=w354:dbl)
          n339 = local read "FWD"() -> (w352:dbl)
          n340 = local read "STR"() -> (w351:dbl)
          n341 = Cosine(x=w359) -> (cos(x)=w367:dbl)
          n342 = Sine(x=w354) -> (sin(x)=w366:dbl)
          n343 = Multiply(x=w352, y=w366) -> (x*y=w353:dbl)
          n344 = Multiply(x=w351, y=w367) -> (x*y=w365:dbl)
          n345 = Add(x=w365, y=w353) -> (x+y=w364:dbl)
          n346 = local write "STR"(w364) -> ()
        }
        frame #3 {
          n347 = local read "temp"() -> (w368:dbl)
          n348 = local write "FWD"(w368) -> ()
        }
        frame #4 {
          n349 = local read "R"() -> (w372:dbl)
          n350 = local read "L"() -> (w371:dbl)
          n351 = local read "R"() -> (w379:dbl)
          n352 = local read "L"() -> (w380:dbl)
          n353 = local read "W"() -> (w384:dbl)
          n354 = local read "R"() -> (w385:dbl)
          n355 = local read "W"() -> (w395:dbl)
          n356 = local read "R"() -> (w394:dbl)
          n357 = Divide(x=w371, y=w372) -> (x/y=w373:dbl)
          n358 = local read "RCW"() -> (w370:dbl)
          n359 = Divide(x=w380, y=w379) -> (x/y=w378:dbl)
          n360 = local read "RCW"() -> (w381:dbl)
          n361 = Divide(x=w384, y=w385) -> (x/y=w386:dbl)
          n362 = local read "RCW"() -> (w383:dbl)
          n363 = Divide(x=w395, y=w394) -> (x/y=w393:dbl)
          n364 = local read "RCW"() -> (w396:dbl)
          n365 = local read "STR"() -> (w369:dbl)
          n366 = local read "STR"() -> (w382:dbl)
          n367 = local read "FWD"() -> (w389:dbl)
          n368 = local read "FWD"() -> (w390:dbl)
          n369 = Multiply(x=w370, y=w373) -> (x*y=w374:dbl)
          n370 = Multiply(x=w381, y=w378) -> (x*y=w377:dbl)
          n371 = Multiply(x=w383, y=w386) -> (x*y=w387:dbl)
          n372 = Multiply(x=w396, y=w393) -> (x*y=w392:dbl)
          n373 = Subtract(x=w369, y=w374) -> (x-y=w375:dbl)
          n374 = Add(x=w382, y=w377) -> (x+y=w376:dbl)
          n375 = Subtract(x=w389, y=w387) -> (x-y=w388:dbl)
          n376 = Add(x=w390, y=w392) -> (x+y=w391:dbl)
          n377 = local write "A"(w375) -> ()
          n378 = local write "B"(w376) -> ()
          n379 = local write "C"(w388) -> ()
          n380 = local write "D"(w391) -> ()
        }
        frame #5 {
          n381 = local read "A"() -> (w409:dbl)
          n382 = local read "A"() -> (w419:dbl)
          n383 = local read "B"() -> (w408:dbl)
          n384 = local read "D"() -> (w407:dbl)
          n385 = local read "D"() -> (w410:dbl)
          n386 = local read "C"() -> (w418:dbl)
          n387 = local read "B"() -> (w397:dbl)
          n388 = local read "C"() -> (w398:dbl)
          n389 = Square(x=w408) -> (x^2=w406:dbl)
          n390 = Square(x=w407) -> (x^2=w405:dbl)
          n391 = Square(x=w409) -> (x^2=w411:dbl)
          n392 = Square(x=w410) -> (x^2=w412:dbl)
          n393 = Square(x=w419) -> (x^2=w420:dbl)
          n394 = Square(x=w418) -> (x^2=w417:dbl)
          n395 = Square(x=w397) -> (x^2=w399:dbl)
          n396 = Square(x=w398) -> (x^2=w400:dbl)
          n397 = Add(x=w406, y=w405) -> (x+y=w404:dbl)
          n398 = Add(x=w411, y=w412) -> (x+y=w413:dbl)
          n399 = Add(x=w420, y=w417) -> (x+y=w416:dbl)
          n400 = Add(x=w399, y=w400) -> (x+y=w401:dbl)
          n401 = Square Root(x=w404) -> (sqrt(x)=w403:dbl)
          n402 = Square Root(x=w413) -> (sqrt(x)=w414:dbl)
          n403 = Square Root(x=w416) -> (sqrt(x)=w415:dbl)
          n404 = Square Root(x=w401) -> (sqrt(x)=w402:dbl)
          n405 = local write "Temp Speed2"(w414) -> ()
          n406 = local write "Temp Speed3"(w415) -> ()
          n407 = local write "Temp Speed1"(w403) -> ()
          n408 = local write "Temp Speed0"(w402) -> ()
        }
        frame #6 {
          n409 = local read "D"() -> (w445:dbl)
          n410 = local read "A"() -> (w446:dbl)
          n411 = local read "C"() -> (w447:dbl)
          n412 = local read "D"() -> (w443:dbl)
          n413 = local read "B"() -> (w444:dbl)
          n414 = local read "C"() -> (w441:dbl)
          n415 = local read "A"() -> (w448:dbl)
          n416 = local read "B"() -> (w442:dbl)
          n417 = Divide(x=180.0, y=3.141592653589793) -> (x/y=w433:dbl)
          n418 = Divide(x=180.0, y=3.141592653589793) -> (x/y=w436:dbl)
          n419 = Divide(x=180.0, y=3.141592653589793) -> (x/y=w430:dbl)
          n420 = Divide(x=180.0, y=3.141592653589793) -> (x/y=w439:dbl)
          n421 = Inverse Tangent (2 Input)(1:w444, 2:w443) -> (0:w434:dbl)
          n422 = Inverse Tangent (2 Input)(1:w446, 2:w445) -> (0:w435:dbl)
          n423 = Inverse Tangent (2 Input)(1:w442, 2:w441) -> (0:w429:dbl)
          n424 = Inverse Tangent (2 Input)(1:w448, 2:w447) -> (0:w440:dbl)
          n425 = Multiply(x=w434, y=w433) -> (x*y=w432:dbl)
          n426 = Multiply(x=w435, y=w436) -> (x*y=w437:dbl)
          n427 = Multiply(x=w429, y=w430) -> (x*y=w431:dbl)
          n428 = Multiply(x=w440, y=w439) -> (x*y=w438:dbl)
          n429 = local write "Temp Turn1"(w432) -> ()
          n430 = local write "Temp Turn2"(w437) -> ()
          n431 = local write "Temp Turn0"(w431) -> ()
          n432 = local write "Temp Turn3"(w438) -> ()
        }
        frame #7 {
          n433 = local read "Temp Speed0"() -> (w450:dbl)
          n434 = local read "Temp Speed1"() -> (w451:dbl)
          n435 = local read "Temp Speed2"() -> (w452:dbl)
          n436 = Max & Min(x=w450, y=w451) -> (max(x,y)=w453:dbl)  [unwired: 1 out]
          n437 = local read "Temp Speed3"() -> (w455:dbl)
          n438 = Max & Min(x=w453, y=w452) -> (max(x,y)=w454:dbl)  [unwired: 1 out]
          n439 = Max & Min(x=w454, y=w455) -> (max(x,y)=w457:dbl)  [unwired: 1 out]
          n440 = Greater?(x=w457, y=1.0) -> (0:w456:bool)
          n441 = case shown="True" w456 {
            tunnel: w457 -> [_ w469]
            frame False {
              n442 = local read "Temp Speed0"() -> (w461:dbl)
              n443 = local read "Temp Speed1"() -> (w460:dbl)
              n444 = local read "Temp Speed2"() -> (w459:dbl)
              n445 = local read "Temp Speed3"() -> (w458:dbl)
              n446 = local write "Speed2"(w459) -> ()
              n447 = local write "Speed0"(w461) -> ()
              n448 = local write "Speed1"(w460) -> ()
              n449 = local write "Speed3"(w458) -> ()
            }
            frame True {
              n450 = local read "Temp Speed0"() -> (w470:dbl)
              n451 = local read "Temp Speed1"() -> (w466:dbl)
              n452 = local read "Temp Speed3"() -> (w468:dbl)
              n453 = local read "Temp Speed2"() -> (w467:dbl)
              n454 = Divide(x=w467, y=w469) -> (x/y=w463:dbl)
              n455 = Divide(x=w466, y=w469) -> (x/y=w464:dbl)
              n456 = Divide(x=w468, y=w469) -> (x/y=w462:dbl)
              n457 = Divide(x=w470, y=w469) -> (x/y=w465:dbl)
              n458 = local write "Speed2"(w463) -> ()
              n459 = local write "Speed0"(w465) -> ()
              n460 = local write "Speed1"(w464) -> ()
              n461 = local write "Speed3"(w462) -> ()
            }
          }
        }
      }
      n462 = stacked-sequence {
        frame #0 {
          # "Preparation for Swerve-n-Turn"
          # "Convert 0 to -/+180 to 0-4096\nfor steering position"
          # "Convert 0-360 Degrees\nto -180 (CCW) to \n+180 (CW)"
          # "Convert Joystick\nRadians to 0-360\nDegrees"
          n463 = local read "Temp Turn0"() -> (w613:dbl)
          n464 = Greater?(x=w613, y=180.0) -> (0:w626:bool)
          n465 = Subtract(x=360.0, y=w613) -> (x-y=w623:dbl)
          n466 = Multiply(x=w613, y=-1.0) -> (x*y=w625:dbl)
          n467 = Select(t=w623, s=w626, f=w625) -> (s? t:f=w614:dbl)
          n468 = local write "+-180"(w614) -> ()
          n469 = expression code="x*(2048/180)"(w613) -> (w616:dbl)
          n470 = expression code="-2048/180"(0.0) -> (w619:dbl)
          n471 = Greater Or Equal To 0?(x=w613) -> (x >= 0?=w621:bool)
          n472 = Multiply(x=w613, y=w619) -> (x*y=w615:dbl)
          n473 = Subtract(x=4096.0, y=w616) -> (x-y=w617:dbl)
          n474 = Select(t=w617, s=w621, f=w615) -> (s? t:f=w612:dbl)
          n475 = local write "Turn0"(w612) -> ()
        }
        frame #1 {
          # "Preparation for Swerve-n-Turn"
          # "Convert 0 to -/+180 to 0-4096\nfor steering position"
          # "Convert 0-360 Degrees\nto -180 (CCW) to \n+180 (CW)"
          # "Convert Joystick\nRadians to 0-360\nDegrees"
          n476 = local read "Temp Turn1"() -> (w629:dbl)
          n477 = Greater?(x=w629, y=180.0) -> (0:w642:bool)
          n478 = Subtract(x=360.0, y=w629) -> (x-y=w639:dbl)
          n479 = Multiply(x=w629, y=-1.0) -> (x*y=w641:dbl)
          n480 = Select(t=w639, s=w642, f=w641) -> (s? t:f=w630:dbl)
          n481 = local write "+-180"(w630) -> ()
          n482 = expression code="x*(2048/180)"(w629) -> (w632:dbl)
          n483 = expression code="-2048/180"(0.0) -> (w635:dbl)
          n484 = Greater Or Equal To 0?(x=w629) -> (x >= 0?=w637:bool)
          n485 = Multiply(x=w629, y=w635) -> (x*y=w631:dbl)
          n486 = Subtract(x=4096.0, y=w632) -> (x-y=w633:dbl)
          n487 = Select(t=w633, s=w637, f=w631) -> (s? t:f=w628:dbl)
          n488 = local write "Turn1"(w628) -> ()
        }
        frame #2 {
          # "Preparation for Swerve-n-Turn"
          # "Convert 0 to -/+180 to 0-4096\nfor steering position"
          # "Convert 0-360 Degrees\nto -180 (CCW) to \n+180 (CW)"
          # "Convert Joystick\nRadians to 0-360\nDegrees"
          n489 = local read "Temp Turn2"() -> (w645:dbl)
          n490 = Greater?(x=w645, y=180.0) -> (0:w658:bool)
          n491 = Subtract(x=360.0, y=w645) -> (x-y=w655:dbl)
          n492 = Multiply(x=w645, y=-1.0) -> (x*y=w657:dbl)
          n493 = Select(t=w655, s=w658, f=w657) -> (s? t:f=w646:dbl)
          n494 = local write "+-180"(w646) -> ()
          n495 = expression code="x*(2048/180)"(w645) -> (w648:dbl)
          n496 = expression code="-2048/180"(0.0) -> (w651:dbl)
          n497 = Greater Or Equal To 0?(x=w645) -> (x >= 0?=w653:bool)
          n498 = Multiply(x=w645, y=w651) -> (x*y=w647:dbl)
          n499 = Subtract(x=4096.0, y=w648) -> (x-y=w649:dbl)
          n500 = Select(t=w649, s=w653, f=w647) -> (s? t:f=w644:dbl)
          n501 = local write "Turn2"(w644) -> ()
        }
        frame #3 {
          # "Preparation for Swerve-n-Turn"
          # "Convert 0 to -/+180 to 0-4096\nfor steering position"
          # "Convert 0-360 Degrees\nto -180 (CCW) to \n+180 (CW)"
          # "Convert Joystick\nRadians to 0-360\nDegrees"
          n502 = local read "Temp Turn3"() -> (w661:dbl)
          n503 = Greater?(x=w661, y=180.0) -> (0:w674:bool)
          n504 = Subtract(x=360.0, y=w661) -> (x-y=w671:dbl)
          n505 = Multiply(x=w661, y=-1.0) -> (x*y=w673:dbl)
          n506 = Select(t=w671, s=w674, f=w673) -> (s? t:f=w662:dbl)
          n507 = local write "+-180"(w662) -> ()
          n508 = expression code="x*(2048/180)"(w661) -> (w664:dbl)
          n509 = expression code="-2048/180"(0.0) -> (w667:dbl)
          n510 = Greater Or Equal To 0?(x=w661) -> (x >= 0?=w669:bool)
          n511 = Multiply(x=w661, y=w667) -> (x*y=w663:dbl)
          n512 = Subtract(x=4096.0, y=w664) -> (x-y=w665:dbl)
          n513 = Select(t=w665, s=w669, f=w663) -> (s? t:f=w660:dbl)
          n514 = local write "Turn3"(w660) -> ()
        }
      }
      n515 = stacked-sequence {
        frame #0 {
          n516 = local read "Turn0"() -> (w471:dbl)
          n517 = feedback #3() -> (w472:dbl)  [unwired: 1 in]
          n518 = feedback-in #3(w471) -> ()
          n519 = feedback-in #4(w471) -> ()
          n520 = feedback #4() -> (w487:dbl)  [unwired: 1 in]
          n521 = In Range and Coerce(upper limit=5000.0, x=w471, lower limit=3000.0) -> (In Range?=w477:bool)  [unwired: 1 out]
          n522 = In Range and Coerce(upper limit=1000.0, x=w472, lower limit=-1000.0) -> (In Range?=w478:bool)  [unwired: 1 out]
          n523 = In Range and Coerce(upper limit=1000.0, x=w471, lower limit=-1000.0) -> (In Range?=w482:bool)  [unwired: 1 out]
          n524 = In Range and Coerce(upper limit=5000.0, x=w487, lower limit=3000.0) -> (In Range?=w481:bool)  [unwired: 1 out]
          n525 = And(x=w477, y=w478) -> (x .and. y?=w479:bool)
          n526 = And(x=w482, y=w481) -> (x .and. y?=w480:bool)
          n527 = case shown="True" w479 {
            frame False {
            }
            frame True {
              n528 = local read "Rotate 0"() -> (w489:dbl)
              n529 = Decrement(x=w489) -> (x-1=w488:dbl)
              n530 = local write "Rotate 0"(w488) -> ()
            }
          }
          n531 = case shown="True" w480 {
            frame False {
            }
            frame True {
              n532 = local read "Rotate 0"() -> (w491:dbl)
              n533 = Increment(x=w491) -> (x+1=w490:dbl)
              n534 = local write "Rotate 0"(w490) -> ()
            }
          }
        }
        frame #1 {
          n535 = local read "Turn1"() -> (w492:dbl)
          n536 = feedback #5() -> (w493:dbl)  [unwired: 1 in]
          n537 = feedback-in #5(w492) -> ()
          n538 = feedback-in #6(w492) -> ()
          n539 = feedback #6() -> (w508:dbl)  [unwired: 1 in]
          n540 = In Range and Coerce(upper limit=5000.0, x=w492, lower limit=3000.0) -> (In Range?=w498:bool)  [unwired: 1 out]
          n541 = In Range and Coerce(upper limit=1000.0, x=w493, lower limit=-1000.0) -> (In Range?=w499:bool)  [unwired: 1 out]
          n542 = In Range and Coerce(upper limit=1000.0, x=w492, lower limit=-1000.0) -> (In Range?=w503:bool)  [unwired: 1 out]
          n543 = In Range and Coerce(upper limit=5000.0, x=w508, lower limit=3000.0) -> (In Range?=w502:bool)  [unwired: 1 out]
          n544 = And(x=w498, y=w499) -> (x .and. y?=w500:bool)
          n545 = And(x=w503, y=w502) -> (x .and. y?=w501:bool)
          n546 = case shown="True" w500 {
            frame False {
            }
            frame True {
              n547 = local read "Rotate 1"() -> (w510:dbl)
              n548 = Decrement(x=w510) -> (x-1=w509:dbl)
              n549 = local write "Rotate 1"(w509) -> ()
            }
          }
          n550 = case shown="True" w501 {
            frame False {
            }
            frame True {
              n551 = local read "Rotate 1"() -> (w511:dbl)
              n552 = Increment(x=w511) -> (x+1=w512:dbl)
              n553 = local write "Rotate 1"(w512) -> ()
            }
          }
        }
        frame #2 {
          n554 = local read "Turn2"() -> (w513:dbl)
          n555 = feedback #7() -> (w514:dbl)  [unwired: 1 in]
          n556 = feedback-in #7(w513) -> ()
          n557 = feedback-in #8(w513) -> ()
          n558 = feedback #8() -> (w529:dbl)  [unwired: 1 in]
          n559 = In Range and Coerce(upper limit=5000.0, x=w513, lower limit=3000.0) -> (In Range?=w519:bool)  [unwired: 1 out]
          n560 = In Range and Coerce(upper limit=1000.0, x=w514, lower limit=-1000.0) -> (In Range?=w520:bool)  [unwired: 1 out]
          n561 = In Range and Coerce(upper limit=1000.0, x=w513, lower limit=-1000.0) -> (In Range?=w524:bool)  [unwired: 1 out]
          n562 = In Range and Coerce(upper limit=5000.0, x=w529, lower limit=3000.0) -> (In Range?=w523:bool)  [unwired: 1 out]
          n563 = And(x=w519, y=w520) -> (x .and. y?=w521:bool)
          n564 = And(x=w524, y=w523) -> (x .and. y?=w522:bool)
          n565 = case shown="True" w521 {
            frame False {
            }
            frame True {
              n566 = local read "Rotate 2"() -> (w531:dbl)
              n567 = Decrement(x=w531) -> (x-1=w530:dbl)
              n568 = local write "Rotate 2"(w530) -> ()
            }
          }
          n569 = case shown="True" w522 {
            frame False {
            }
            frame True {
              n570 = local read "Rotate 2"() -> (w532:dbl)
              n571 = Increment(x=w532) -> (x+1=w533:dbl)
              n572 = local write "Rotate 2"(w533) -> ()
            }
          }
        }
        frame #3 {
          n573 = local read "Turn3"() -> (w534:dbl)
          n574 = feedback #9() -> (w535:dbl)  [unwired: 1 in]
          n575 = feedback-in #9(w534) -> ()
          n576 = feedback-in #10(w534) -> ()
          n577 = feedback #10() -> (w550:dbl)  [unwired: 1 in]
          n578 = In Range and Coerce(upper limit=5000.0, x=w534, lower limit=3000.0) -> (In Range?=w540:bool)  [unwired: 1 out]
          n579 = In Range and Coerce(upper limit=1000.0, x=w535, lower limit=-1000.0) -> (In Range?=w541:bool)  [unwired: 1 out]
          n580 = In Range and Coerce(upper limit=1000.0, x=w534, lower limit=-1000.0) -> (In Range?=w545:bool)  [unwired: 1 out]
          n581 = In Range and Coerce(upper limit=5000.0, x=w550, lower limit=3000.0) -> (In Range?=w544:bool)  [unwired: 1 out]
          n582 = And(x=w540, y=w541) -> (x .and. y?=w542:bool)
          n583 = And(x=w545, y=w544) -> (x .and. y?=w543:bool)
          n584 = case shown="True" w543 {
            frame False {
            }
            frame True {
              n585 = local read "Rotate 3"() -> (w553:dbl)
              n586 = Increment(x=w553) -> (x+1=w554:dbl)
              n587 = local write "Rotate 3"(w554) -> ()
            }
          }
          n588 = case shown="True" w542 {
            frame False {
            }
            frame True {
              n589 = local read "Rotate 3"() -> (w552:dbl)
              n590 = Decrement(x=w552) -> (x-1=w551:dbl)
              n591 = local write "Rotate 3"(w551) -> ()
            }
          }
        }
      }
      n592 = case shown="True" TRUE {
        frame False {
        }
        frame True {
          w578 = T3 1 items=["PercentOutput"=0, "Position"=1, "Velocity"=2, "Current"=3, "Follower"=5, "MotionProfile"=6, "MotionMagic"=7, "MotionMagicArc"=8, "MotionProfileArc"=10, "Disabled"=15] ("Control Mode")
          n593 = local read "Rotate 3"() -> (w563:dbl)
          n594 = local read "Rotate 2"() -> (w566:dbl)
          n595 = local read "Rotate 0"() -> (w572:dbl)
          n596 = local read "Rotate 1"() -> (w569:dbl)
          n597 = local read "Turn3"() -> (w562:dbl)
          n598 = local read "Turn2"() -> (w567:dbl)
          n599 = local read "Turn0"() -> (w579:dbl)
          n600 = local read "Turn1"() -> (w568:dbl)
          n601 = Multiply(x=w563, y=4096.0) -> (x*y=w555:dbl)
          n602 = Multiply(x=w566, y=4096.0) -> (x*y=w556:dbl)
          n603 = Multiply(x=w572, y=4096.0) -> (x*y=w558:dbl)
          n604 = Multiply(x=w569, y=4096.0) -> (x*y=w557:dbl)
          n605 = Add(x=w562, y=w555) -> (x+y=w559:dbl)
          n606 = Add(x=w567, y=w556) -> (x+y=w560:dbl)
          n607 = Add(x=w579, y=w558) -> (x+y=w573:dbl)
          n608 = Add(x=w568, y=w557) -> (x+y=w561:dbl)
          n609 = local read "Speed2"() -> (w589:dbl)
          n610 = local read "Speed0"() -> (w591:dbl)
          n611 = local read "Speed1"() -> (w590:dbl)
          n612 = local read "Speed3"() -> (w588:dbl)
          n613 = call "CTRE_Phoenix_MotorControl_RefNumRegistryGet.vi"("refnum name"="Turn0") -> ("error out"=w587:errorcluster, "PhoenixMotorControlDevRef"=w586:T4)  [unwired: 9 in]
          n614 = call "CTRE_Phoenix_MotorControl_RefNumRegistryGet.vi"("refnum name"="Turn1") -> ("error out"=w580:errorcluster, "PhoenixMotorControlDevRef"=w581:T4)  [unwired: 9 in]
          n615 = call "CTRE_Phoenix_MotorControl_RefNumRegistryGet.vi"("refnum name"="Turn2") -> ("error out"=w585:errorcluster, "PhoenixMotorControlDevRef"=w584:T4)  [unwired: 9 in]
          n616 = call "CTRE_Phoenix_MotorControl_RefNumRegistryGet.vi"("refnum name"="Turn3") -> ("error out"=w583:errorcluster, "PhoenixMotorControlDevRef"=w582:T4)  [unwired: 9 in]
          n617 = call "CTRE_Phoenix_MotorControl_RefNumRegistryGet.vi"("refnum name"="Drive0") -> ("PhoenixMotorControlDevRef"=w596:T4)  [unwired: 9 in, 1 out]
          n618 = call "CTRE_Phoenix_MotorControl_RefNumRegistryGet.vi"("refnum name"="Drive1") -> ("PhoenixMotorControlDevRef"=w597:T4)  [unwired: 9 in, 1 out]
          n619 = call "CTRE_Phoenix_MotorControl_RefNumRegistryGet.vi"("refnum name"="Drive2") -> ("PhoenixMotorControlDevRef"=w598:T4)  [unwired: 9 in, 1 out]
          n620 = call "CTRE_Phoenix_MotorControl_RefNumRegistryGet.vi"("refnum name"="Drive3") -> ("PhoenixMotorControlDevRef"=w599:T4)  [unwired: 9 in, 1 out]
          n621 = call "CTRE_Phoenix_MotorControl_Set.vi"("error in (no error)"=w580, "Output"=w561, "Control Mode"=w578, "PhoenixMotorControlDevRef"=w581) -> ()  [unwired: 6 in, 2 out]
          n622 = call "CTRE_Phoenix_MotorControl_Set.vi"("error in (no error)"=w585, "Output"=w560, "Control Mode"=w578, "PhoenixMotorControlDevRef"=w584) -> ()  [unwired: 6 in, 2 out]
          n623 = call "CTRE_Phoenix_MotorControl_Set.vi"("error in (no error)"=w583, "Output"=w559, "Control Mode"=w578, "PhoenixMotorControlDevRef"=w582) -> ()  [unwired: 6 in, 2 out]
          n624 = call "CTRE_Phoenix_MotorControl_Set.vi"("error in (no error)"=w587, "Output"=w573, "Control Mode"=w578, "PhoenixMotorControlDevRef"=w586) -> ()  [unwired: 6 in, 2 out]
          n625 = call <vilib>:"WPI_MotorControlSetOutput.vi"("Output"=w591, "MotorControlDevRef"=w596) -> ()  [unwired: 7 in, 3 out]
          n626 = call <vilib>:"WPI_MotorControlSetOutput.vi"("Output"=w590, "MotorControlDevRef"=w597) -> ()  [unwired: 7 in, 3 out]
          n627 = call <vilib>:"WPI_MotorControlSetOutput.vi"("Output"=w589, "MotorControlDevRef"=w598) -> ()  [unwired: 7 in, 3 out]
          n628 = call <vilib>:"WPI_MotorControlSetOutput.vi"("Output"=w588, "MotorControlDevRef"=w599) -> ()  [unwired: 7 in, 3 out]
        }
      }
    }
  }
